vi "NanotecSMCPD.ProcCases.vi"(0 "i ref in":refnum<vi>, 1 "selector":string, 2 "Data":T1, 3 "call cluster":T2={"Object"="", "Selector"="", "CallType"=enum."synchronous", "Async Object"="", "Async Selector"="", "Data Descriptor"="", "Data"=[], "Error #"=0, "Expire"=0}, 5 "error in (no error)":errorcluster) -> (14 "i ref out":refnum<vi>, 17 "answer cluster":T2={"Object"="", "Selector"="", "CallType"=enum."synchronous", "Async Object"="", "Async Selector"="", "Data Descriptor"="", "Data"=[], "Error #"=0, "Expire"=0}, 19 "error out":errorcluster)   [LabVIEW 2014, in "NanotecSMCPD.lvlib"]
doc: "This method is called by a process from within the default case in the event loop. The methods of a class that are linked to events will be called from THIS method. Add your code here."
uses:
  NanotecSMCPD.lvlib
  CS_Core/CSSystem/CoreDefs/CoreDefs.call_type.ctl
  CS_Core/BaseProcess/BaseProcess.descriptor string definition.ctl
  CS_Core/CSSystem/CoreDefs/CoreDefs.rawDataType.ctl
  CS_Core/CSApplicationBaseClasses/MotorBase/MotorBase.statusType.ctl
  CS_Core/CSSystem/CoreLib/CoreLib.string 2 byte array.vi
  CS_Core/CSSystem/CoreLib/CoreLib.short 2 byte array.vi
  CS_Core/CSSystem/CoreLib/CoreLib.byte array 2 int.vi
  CS_Core/CSSystem/CoreLib/CoreLib.int 2 byte array.vi
  CS_Core/CSSystem/CoreLib/CoreLib.double 2 byte array.vi
  CS_Core/CSSystem/CoreLib/CoreLib.byte array 2 double.vi
  CS_Core/CSSystem/CoreLib/CoreLib.byte array 2 short.vi
  CS_Core/CSSystem/CoreLib/CoreLib.lvlib
  CS_Core/BaseProcess/BaseProcess.lvlib
  CS_Core/CSApplicationBaseClasses/MotorBase/MotorBase.lvlib
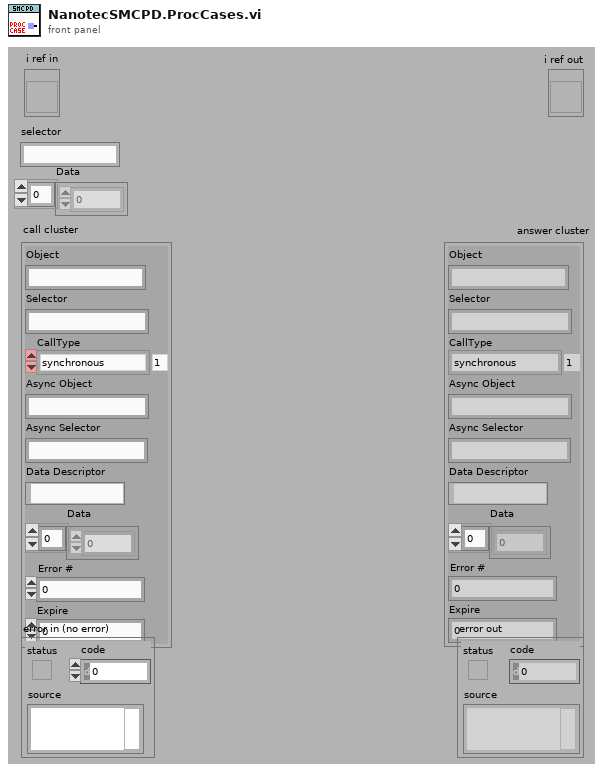
[diagram p1: front panel]
types:
  T1 = typedef "CoreDefs.rawDataType.ctl" = i8[]
  T2 = typedef "CoreDefs.call_type.ctl" = cluster{"Object":string, "Selector":string, "CallType":enum16{"simple", "synchronous", "asynchronous"}, "Async Object":string, "Async Selector":string, "Data Descriptor":T3, "Data":T1, "Error #":i32, "Expire":u32}
  T3 = typedef "BaseProcess.lvlib/BaseProcess.descriptor string definition.ctl" = string
  T4 = typedef "MotorBase.lvlib/MotorBase.statusType.ctl" = u32
  T5 = cluster{"Method":enum16{"MoveRelative", "MoveAbsolute", "Stop"}, "Axis":i32, "Steps":dbl}
  T6 = typedef "NanotecSMCPD.lvlib/NanotecSMCPD.i attribute.ctl" = cluster{"referencing":bool[], "stop":bool[], "AutoHalt ID":i32, "MethodQueue":refnum<queue>, "Referenced1Time?":bool[], "LastCommand ID":i32}
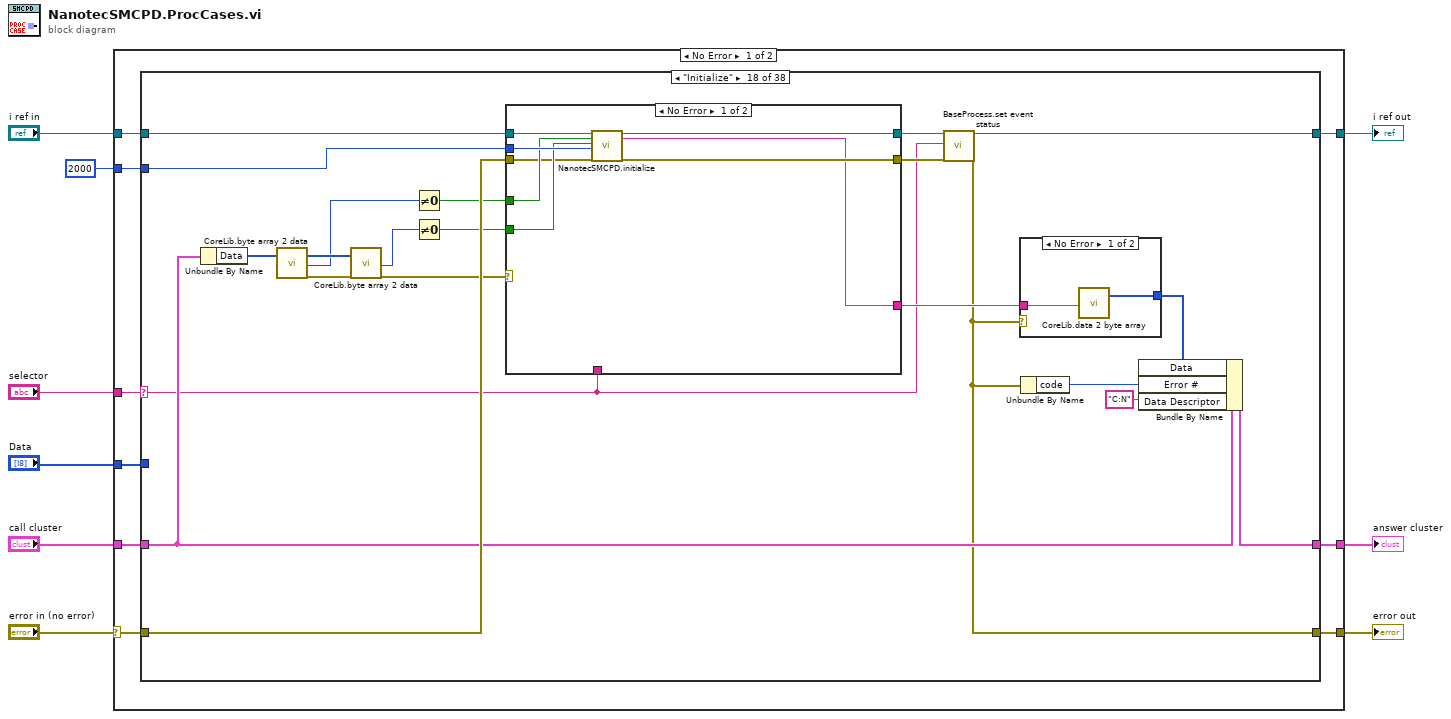
[diagram p0: block diagram]
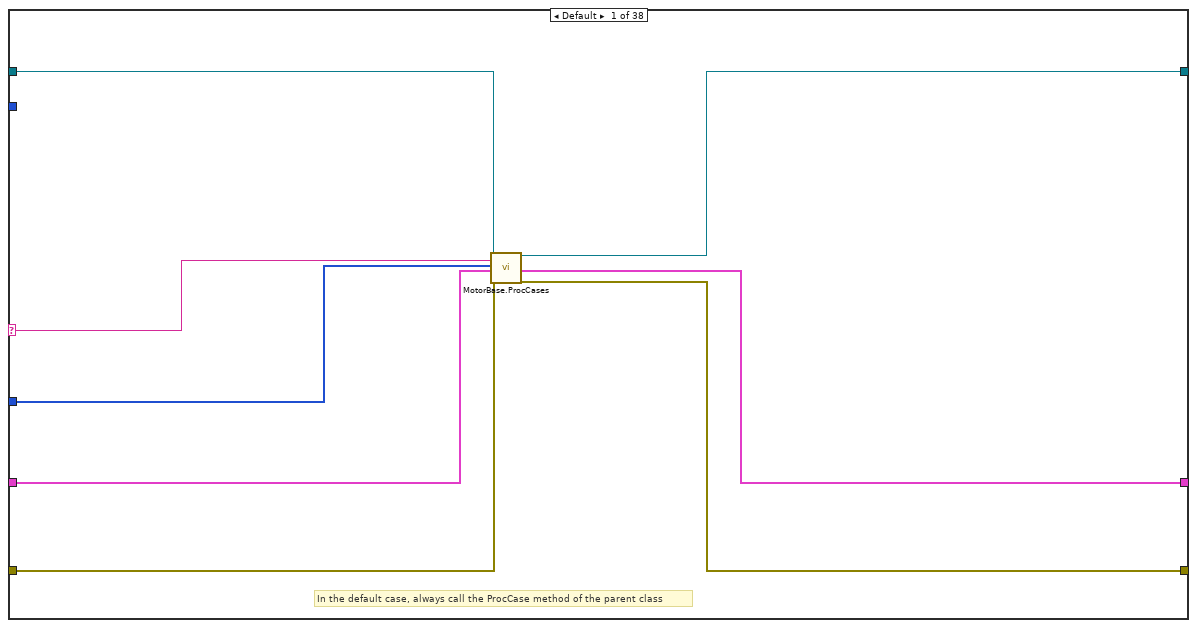
[diagram p2: hidden frame]
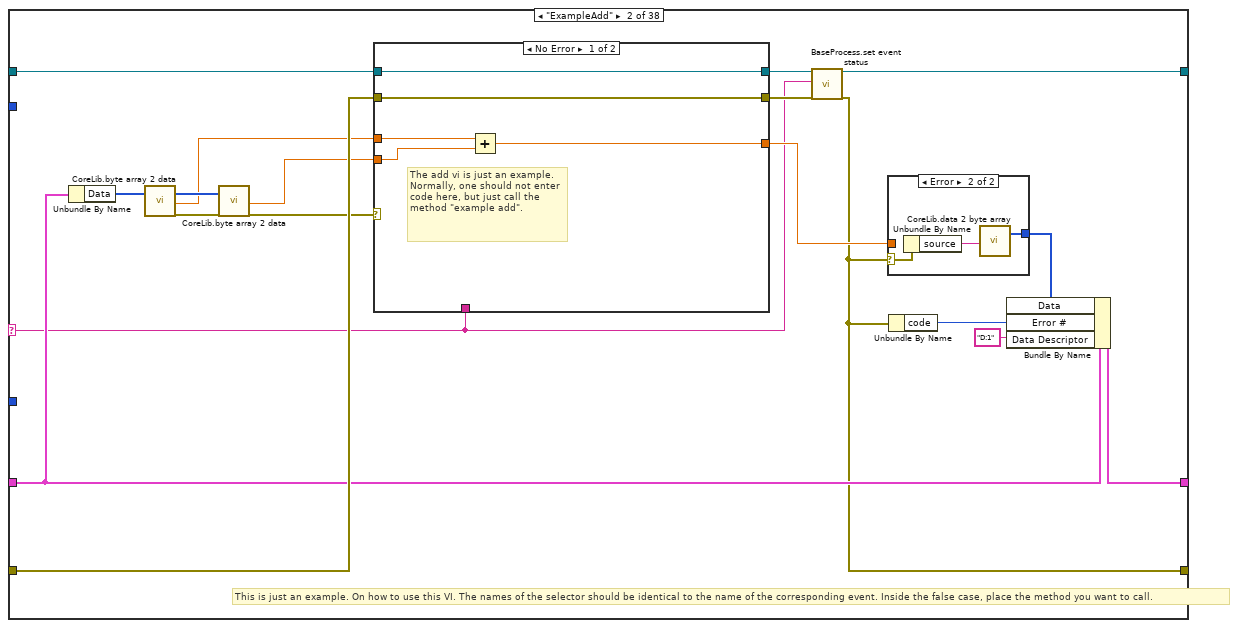
[diagram p3: hidden frame]
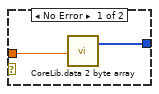
[diagram p4: hidden frame]
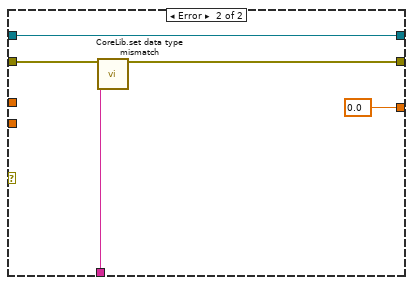
[diagram p5: hidden frame]
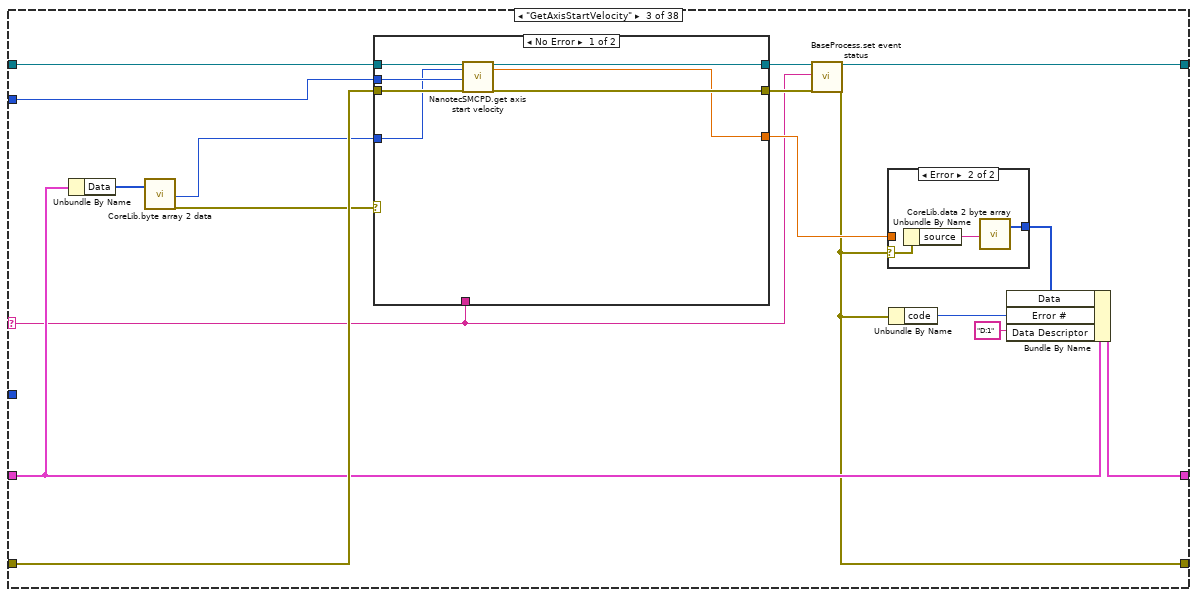
[diagram p6: hidden frame]
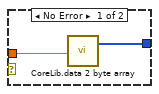
[diagram p7: hidden frame]
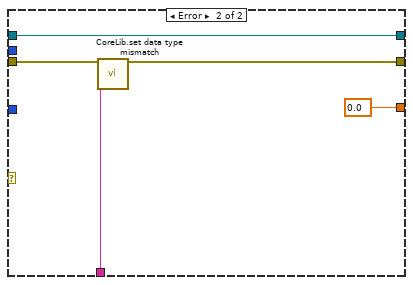
[diagram p8: hidden frame]
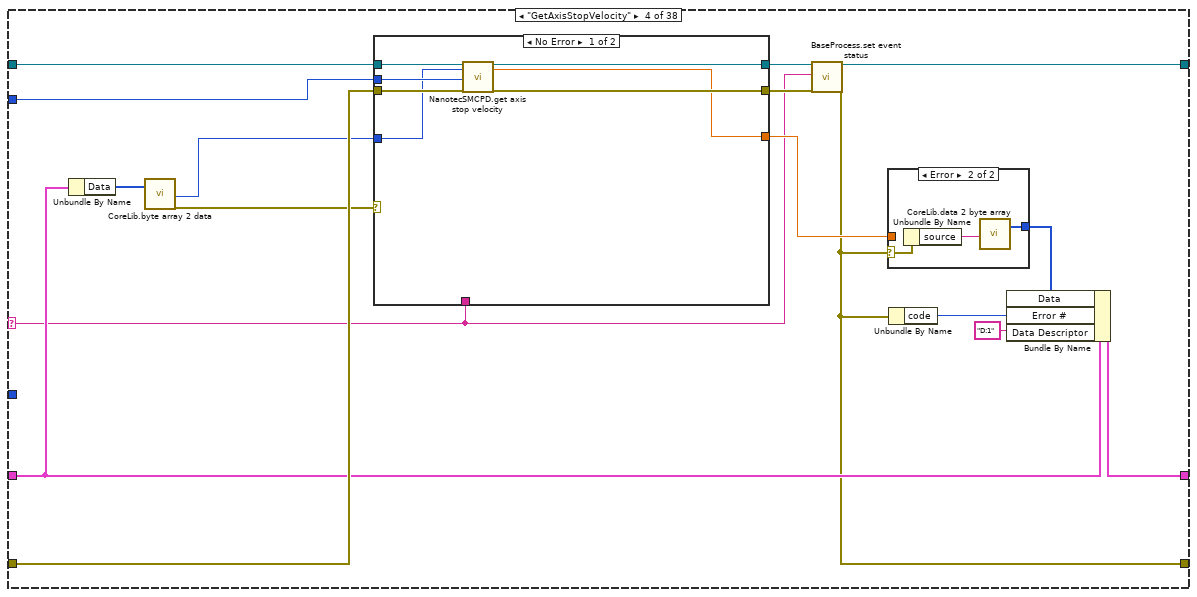
[diagram p9: hidden frame]
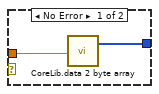
[diagram p10: hidden frame]
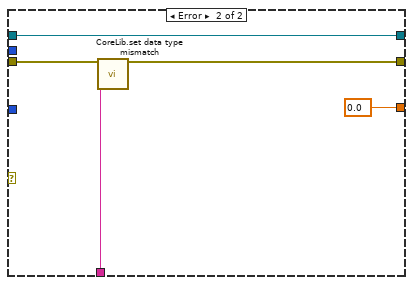
[diagram p11: hidden frame]
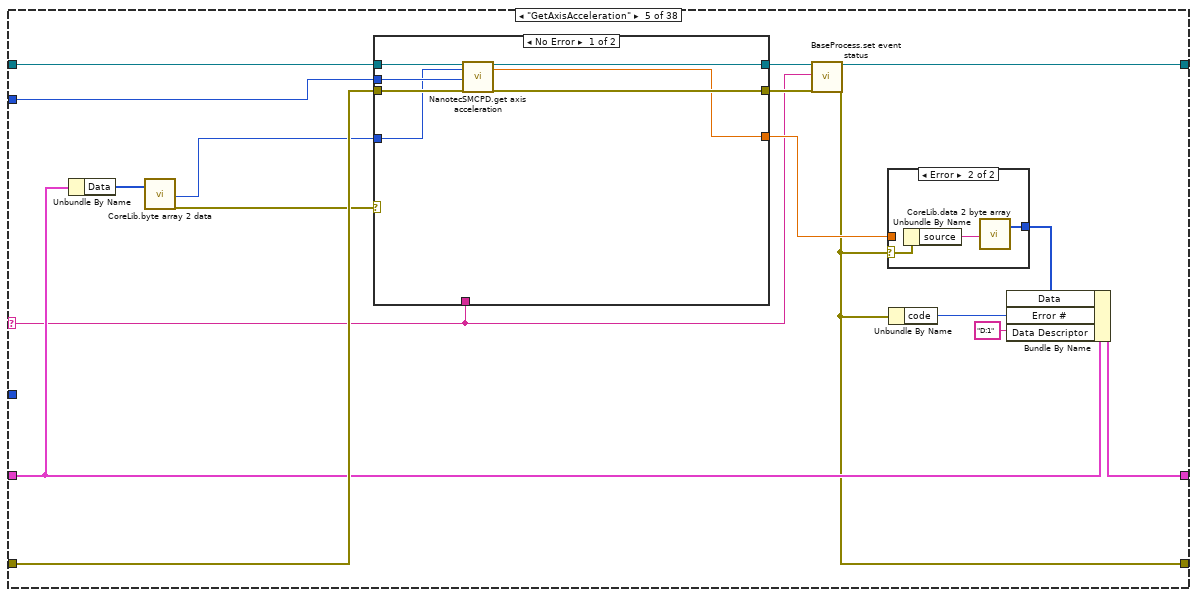
[diagram p12: hidden frame]
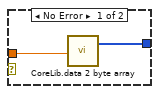
[diagram p13: hidden frame]
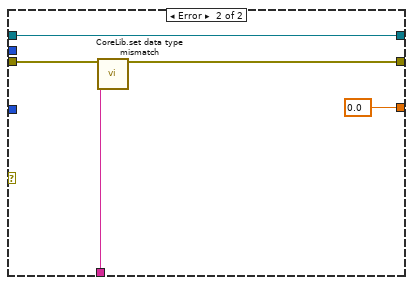
[diagram p14: hidden frame]
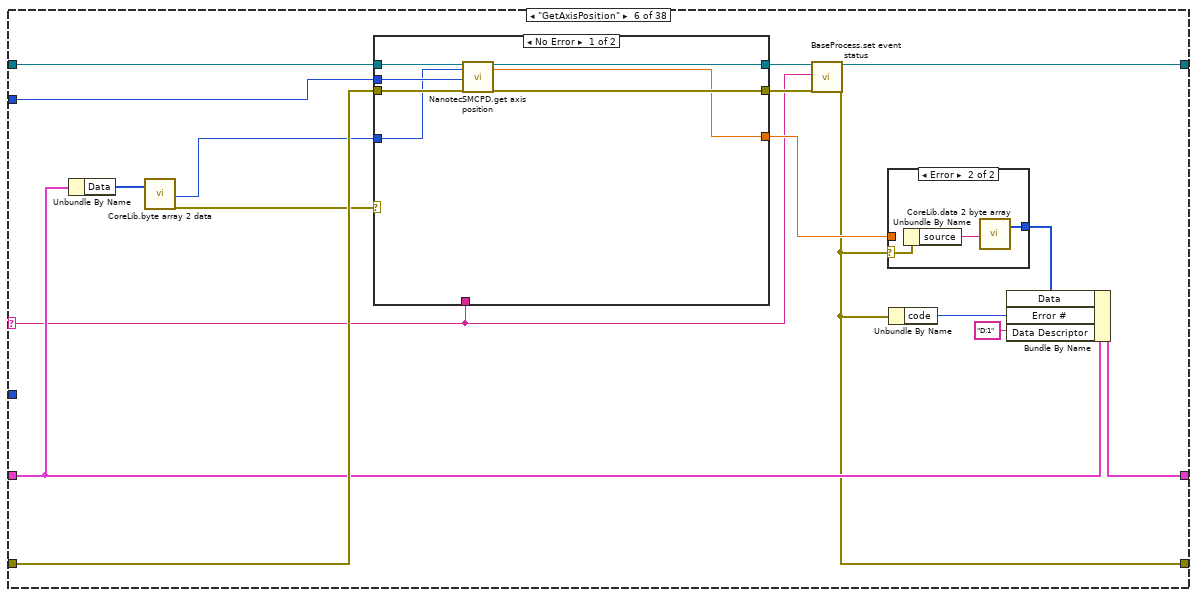
[diagram p15: hidden frame]
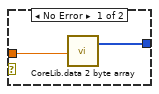
[diagram p16: hidden frame]
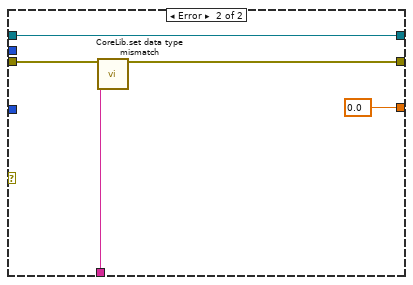
[diagram p17: hidden frame]
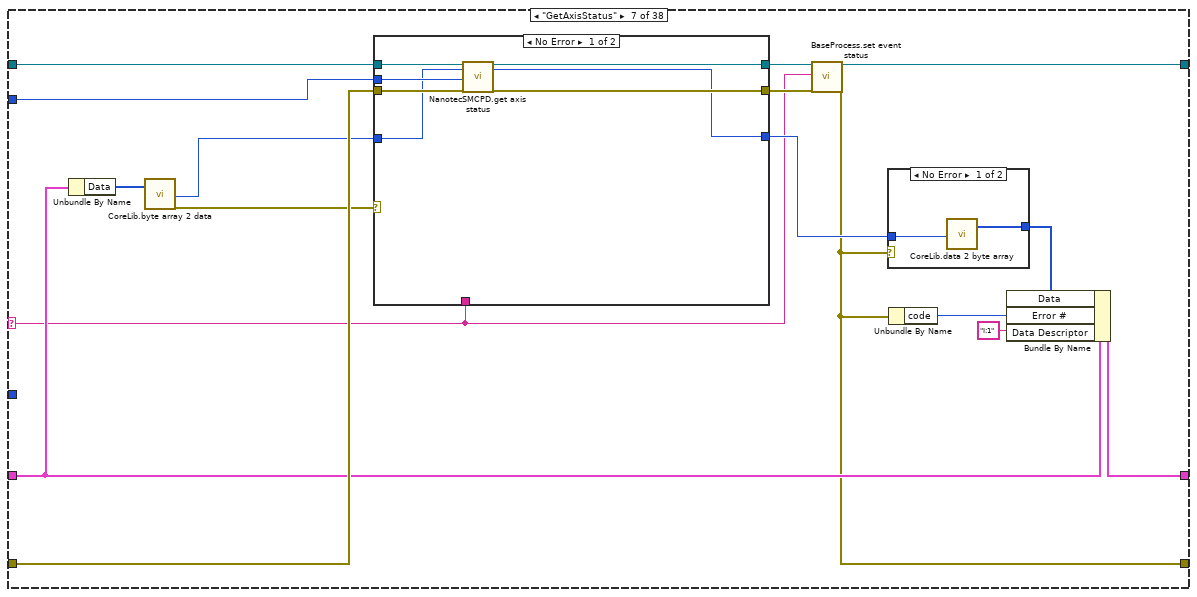
[diagram p18: hidden frame]
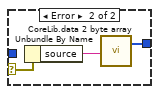
[diagram p19: hidden frame]
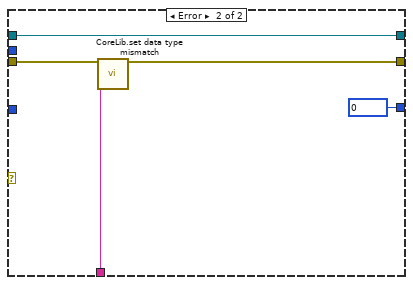
[diagram p20: hidden frame]
diagram:
  n1 = case shown="No Error" "error in (no error)" {
    selector: "error in (no error)" -> [w11 w1067]
    tunnel: "selector" -> [w18 _]
    tunnel: [w17 w1068] -> w8
    tunnel: "Data" -> [w16 _]
    tunnel: "call cluster" -> [w15 w1068]
    tunnel: "i ref in" -> [w14 w1069]
    tunnel: [w13 w1069] -> w4
    tunnel: [w12 w1067] -> w3
    tunnel: 2000 ("ms timeout (10000)") -> [w10 _]
    frame No Error {
      n2 = case shown="\"Initialize\"" w18 {
        selector: w18 -> [w21 w35 w67 w101 w135 w169 w203 w236 w262 w292 w320 w351 w383 w415 w447 w479 w516 w556 w589 w620 w651 w682 w713 w749 w787 w809 w831 w853 w875 w896 w914 w932 w946 w961 w978 w1004 w1018 w1058]
        tunnel: w16 -> [w19 _ _ _ _ _ _ _ _ _ _ _ _ _ _ _ _ _ _ _ _ _ _ _ _ _ _ _ _ _ _ _ _ _ _ _ _ _]
        tunnel: w14 -> [w20 w45 w77 w111 w145 w179 w213 w245 w260 w301 w329 w360 w392 w424 w456 w488 w525 w566 w598 w629 w660 w691 w722 w758 w796 w818 w840 w862 w884 w905 w923 w941 w955 w970 w987 w998 w1023 w1056]
        tunnel: [w26 w34 w66 w100 w134 w168 w202 w235 w259 w291 w319 w350 w382 w414 w446 w478 w515 w555 w588 w619 w650 w681 w712 w748 w786 w808 w830 w852 w874 w895 w913 w931 w945 w960 w977 w1003 w1027 w1057] -> w13
        tunnel: w15 -> [w22 w41 w73 w107 w141 w175 w209 w242 w263 w298 w326 w357 w389 w421 w453 w485 w522 w562 w595 w626 w657 w688 w719 w755 w793 w815 w837 w859 w881 w902 w920 w938 w952 w967 w984 w1010 w1021 w1062]
        tunnel: [w23 w40 w72 w106 w140 w174 w208 w241 w264 w297 w325 w356 w388 w420 w452 w484 w521 w561 w594 w625 w656 w687 w718 w754 w792 w814 w836 w858 w880 w901 w919 w937 w951 w966 w983 w1009 w1032 w1061] -> w17
        tunnel: w11 -> [w25 w44 w76 w110 w144 w178 w212 w244 w266 w300 w328 w359 w391 w423 w455 w487 w524 w565 w597 w628 w659 w690 w721 w757 w795 w817 w839 w861 w883 w904 w922 w940 w954 w969 w986 w995 w1019 w1053]
        tunnel: [w24 w36 w68 w102 w136 w170 w204 w237 w265 w293 w321 w352 w384 w416 w448 w480 w517 w557 w590 w621 w652 w683 w714 w750 w788 w810 w832 w854 w876 w897 w915 w933 w947 w962 w979 w1005 w1028 w1059] -> w12
        tunnel: w10 -> [_ _ w61 w95 w129 w163 w197 w231 w261 w287 w315 w343 w375 w407 w439 w471 w508 w547 w586 w617 w648 w679 w710 w746 w785 w807 w829 w851 w873 w894 w912 w930 _ w959 w976 w993 w1024 w1052]
        frame Default {
          # "In the default case, always call the ProcCase method of the parent class"
          n3 = call "MotorBase.ProcCases.vi"("i ref in"=w20, "selector"=w21, "Data"=w19, "call cluster"=w22, "error in (no error)"=w25) -> ("i ref out"=w26:refnum<vi>, "answer cluster"=w23:T2, "error out"=w24:errorcluster)  [unwired: 12 in]
        }
        frame "ExampleAdd" {
          # "This is just an example. On how to use this VI. The names of the selector should be identical to the name of the corresponding event. Inside the false case, place the method you want to call."
          n4 = Unbundle By Name(w41) -> ("Data"=w32:T1)
          n5 = call-poly "CoreLib.byte array 2 data.vi"("byteArray"=w32) -> ("byteArray out"=w30:T1, "d64"=w28:dbl, "error out"=w31:errorcluster)  [unwired: 16 in]
          n6 = call-poly "CoreLib.byte array 2 data.vi"("byteArray"=w30, "error in (no error)"=w31) -> ("d64"=w27:dbl, "error out"=w29:errorcluster)  [unwired: 15 in, 1 out]
          n7 = case shown="No Error" w29 {
            tunnel: [w52 w60] -> w38
            tunnel: w45 -> [w52 w60]
            tunnel: w44 -> [w53 w59]
            tunnel: [w53 w58] -> w37
            tunnel: w27 -> [w55 _]
            tunnel: [w54 0.0] -> w43
            tunnel: w35 -> [_ w56]
            tunnel: w28 -> [w51 _]
            frame No Error {
              # "The add vi is just an example. Normally, one should not enter code here, but just call the method \"example add\"."
              n8 = Add(x=w51, y=w55) -> (x+y=w54:dbl)
            }
            frame Error {
              n9 = call "CoreLib.set data type mismatch.vi"("error in (no error)"=w59, "error source"=w56) -> ("error out"=w58:errorcluster)  [unwired: 17 in]
            }
          }
          n10 = call "BaseProcess.set event status.vi"("i ref in"=w38, "EventStatus"=w35, "error in (no error)"=w37) -> ("i ref out"=w34:refnum<vi>, "error out"=w36:errorcluster)  [unwired: 14 in, 1 out]
          n11 = case shown="Error" w36 {
            selector: w36 -> [_ w50]
            tunnel: [w46 w49] -> w39
            tunnel: w43 -> [w47 _]
            frame No Error {
              n12 = call-poly "CoreLib.data 2 byte array.vi"("f64"=w47) -> ("byteArray out"=w46:T1)  [unwired: 18 in]
            }
            frame Error {
              n13 = Unbundle By Name(w50) -> ("source"=w48:string)
              n14 = call-poly "CoreLib.data 2 byte array.vi"("string"=w48) -> ("byteArray out"=w49:T1)  [unwired: 18 in]
            }
          }
          n15 = Unbundle By Name(w36) -> ("code"=w42:i32)
          n16 = Bundle By Name(cluster=w41, "Data"=w39, "Error #"=w42, "Data Descriptor"="D:1") -> (w40:T2)
        }
        frame "GetAxisStartVelocity" {
          n17 = Unbundle By Name(w73) -> ("Data"=w64:T1)
          n18 = call-poly "CoreLib.byte array 2 data.vi"("byteArray"=w64) -> ("i32"=w63:i32, "error out"=w62:errorcluster)  [unwired: 16 in, 1 out]
          n19 = case shown="No Error" w62 {
            tunnel: [w88 w94] -> w70
            tunnel: w77 -> [w89 w94]
            tunnel: w76 -> [w86 w93]
            tunnel: [w87 w92] -> w69
            tunnel: [w83 0.0] -> w75
            tunnel: w67 -> [_ w90]
            tunnel: w63 -> [w84 _]
            tunnel: w61 -> [w85 _]
            frame No Error {
              n20 = call "NanotecSMCPD.get axis start velocity.vi"("i ref in"=w89, "axis"=w84, "ms timeout (10000)"=w85, "error in (no error)"=w86) -> ("i ref out"=w88:refnum<vi>, "startVelocity [unit/s]"=w83:dbl, "error out"=w87:errorcluster)  [unwired: 12 in, 1 out]
            }
            frame Error {
              n21 = call "CoreLib.set data type mismatch.vi"("error in (no error)"=w93, "error source"=w90) -> ("error out"=w92:errorcluster)  [unwired: 17 in]
            }
          }
          n22 = call "BaseProcess.set event status.vi"("i ref in"=w70, "EventStatus"=w67, "error in (no error)"=w69) -> ("i ref out"=w66:refnum<vi>, "error out"=w68:errorcluster)  [unwired: 14 in, 1 out]
          n23 = case shown="Error" w68 {
            selector: w68 -> [_ w82]
            tunnel: [w78 w81] -> w71
            tunnel: w75 -> [w79 _]
            frame No Error {
              n24 = call-poly "CoreLib.data 2 byte array.vi"("f64"=w79) -> ("byteArray out"=w78:T1)  [unwired: 18 in]
            }
            frame Error {
              n25 = Unbundle By Name(w82) -> ("source"=w80:string)
              n26 = call-poly "CoreLib.data 2 byte array.vi"("string"=w80) -> ("byteArray out"=w81:T1)  [unwired: 18 in]
            }
          }
          n27 = Unbundle By Name(w68) -> ("code"=w74:i32)
          n28 = Bundle By Name(cluster=w73, "Data"=w71, "Error #"=w74, "Data Descriptor"="D:1") -> (w72:T2)
        }
        frame "GetAxisStopVelocity" {
          n29 = Unbundle By Name(w107) -> ("Data"=w98:T1)
          n30 = call-poly "CoreLib.byte array 2 data.vi"("byteArray"=w98) -> ("i32"=w97:i32, "error out"=w96:errorcluster)  [unwired: 16 in, 1 out]
          n31 = case shown="No Error" w96 {
            tunnel: [w122 w128] -> w104
            tunnel: w111 -> [w123 w128]
            tunnel: w110 -> [w120 w127]
            tunnel: [w121 w126] -> w103
            tunnel: [w117 0.0] -> w109
            tunnel: w101 -> [_ w124]
            tunnel: w97 -> [w118 _]
            tunnel: w95 -> [w119 _]
            frame No Error {
              n32 = call "NanotecSMCPD.get axis stop velocity.vi"("i ref in"=w123, "axis"=w118, "ms timeout (10000)"=w119, "error in (no error)"=w120) -> ("i ref out"=w122:refnum<vi>, "stopVelocity [unit/s]"=w117:dbl, "error out"=w121:errorcluster)  [unwired: 12 in, 1 out]
            }
            frame Error {
              n33 = call "CoreLib.set data type mismatch.vi"("error in (no error)"=w127, "error source"=w124) -> ("error out"=w126:errorcluster)  [unwired: 17 in]
            }
          }
          n34 = call "BaseProcess.set event status.vi"("i ref in"=w104, "EventStatus"=w101, "error in (no error)"=w103) -> ("i ref out"=w100:refnum<vi>, "error out"=w102:errorcluster)  [unwired: 14 in, 1 out]
          n35 = case shown="Error" w102 {
            selector: w102 -> [_ w116]
            tunnel: [w112 w115] -> w105
            tunnel: w109 -> [w113 _]
            frame No Error {
              n36 = call-poly "CoreLib.data 2 byte array.vi"("f64"=w113) -> ("byteArray out"=w112:T1)  [unwired: 18 in]
            }
            frame Error {
              n37 = Unbundle By Name(w116) -> ("source"=w114:string)
              n38 = call-poly "CoreLib.data 2 byte array.vi"("string"=w114) -> ("byteArray out"=w115:T1)  [unwired: 18 in]
            }
          }
          n39 = Unbundle By Name(w102) -> ("code"=w108:i32)
          n40 = Bundle By Name(cluster=w107, "Data"=w105, "Error #"=w108, "Data Descriptor"="D:1") -> (w106:T2)
        }
        frame "GetAxisAcceleration" {
          n41 = Unbundle By Name(w141) -> ("Data"=w132:T1)
          n42 = call-poly "CoreLib.byte array 2 data.vi"("byteArray"=w132) -> ("i32"=w131:i32, "error out"=w130:errorcluster)  [unwired: 16 in, 1 out]
          n43 = case shown="No Error" w130 {
            tunnel: [w156 w162] -> w138
            tunnel: w145 -> [w157 w162]
            tunnel: w144 -> [w154 w161]
            tunnel: [w155 w160] -> w137
            tunnel: [w151 0.0] -> w143
            tunnel: w135 -> [_ w158]
            tunnel: w131 -> [w152 _]
            tunnel: w129 -> [w153 _]
            frame No Error {
              n44 = call "NanotecSMCPD.get axis acceleration.vi"("i ref in"=w157, "axis"=w152, "ms timeout (10000)"=w153, "error in (no error)"=w154) -> ("i ref out"=w156:refnum<vi>, "acceleration [unit/s^2]"=w151:dbl, "error out"=w155:errorcluster)  [unwired: 12 in, 1 out]
            }
            frame Error {
              n45 = call "CoreLib.set data type mismatch.vi"("error in (no error)"=w161, "error source"=w158) -> ("error out"=w160:errorcluster)  [unwired: 17 in]
            }
          }
          n46 = call "BaseProcess.set event status.vi"("i ref in"=w138, "EventStatus"=w135, "error in (no error)"=w137) -> ("i ref out"=w134:refnum<vi>, "error out"=w136:errorcluster)  [unwired: 14 in, 1 out]
          n47 = case shown="Error" w136 {
            selector: w136 -> [_ w150]
            tunnel: [w146 w149] -> w139
            tunnel: w143 -> [w147 _]
            frame No Error {
              n48 = call-poly "CoreLib.data 2 byte array.vi"("f64"=w147) -> ("byteArray out"=w146:T1)  [unwired: 18 in]
            }
            frame Error {
              n49 = Unbundle By Name(w150) -> ("source"=w148:string)
              n50 = call-poly "CoreLib.data 2 byte array.vi"("string"=w148) -> ("byteArray out"=w149:T1)  [unwired: 18 in]
            }
          }
          n51 = Unbundle By Name(w136) -> ("code"=w142:i32)
          n52 = Bundle By Name(cluster=w141, "Data"=w139, "Error #"=w142, "Data Descriptor"="D:1") -> (w140:T2)
        }
        frame "GetAxisPosition" {
          n53 = Unbundle By Name(w175) -> ("Data"=w166:T1)
          n54 = call-poly "CoreLib.byte array 2 data.vi"("byteArray"=w166) -> ("i32"=w165:i32, "error out"=w164:errorcluster)  [unwired: 16 in, 1 out]
          n55 = case shown="No Error" w164 {
            tunnel: [w190 w196] -> w172
            tunnel: w179 -> [w191 w196]
            tunnel: w178 -> [w188 w195]
            tunnel: [w189 w194] -> w171
            tunnel: [w185 0.0] -> w177
            tunnel: w169 -> [_ w192]
            tunnel: w165 -> [w186 _]
            tunnel: w163 -> [w187 _]
            frame No Error {
              n56 = call "NanotecSMCPD.get axis position.vi"("i ref in"=w191, "axis"=w186, "ms timeout (10000)"=w187, "error in (no error)"=w188) -> ("i ref out"=w190:refnum<vi>, "position [unit]"=w185:dbl, "error out"=w189:errorcluster)  [unwired: 12 in, 1 out]
            }
            frame Error {
              n57 = call "CoreLib.set data type mismatch.vi"("error in (no error)"=w195, "error source"=w192) -> ("error out"=w194:errorcluster)  [unwired: 17 in]
            }
          }
          n58 = call "BaseProcess.set event status.vi"("i ref in"=w172, "EventStatus"=w169, "error in (no error)"=w171) -> ("i ref out"=w168:refnum<vi>, "error out"=w170:errorcluster)  [unwired: 14 in, 1 out]
          n59 = case shown="Error" w170 {
            selector: w170 -> [_ w184]
            tunnel: [w180 w183] -> w173
            tunnel: w177 -> [w181 _]
            frame No Error {
              n60 = call-poly "CoreLib.data 2 byte array.vi"("f64"=w181) -> ("byteArray out"=w180:T1)  [unwired: 18 in]
            }
            frame Error {
              n61 = Unbundle By Name(w184) -> ("source"=w182:string)
              n62 = call-poly "CoreLib.data 2 byte array.vi"("string"=w182) -> ("byteArray out"=w183:T1)  [unwired: 18 in]
            }
          }
          n63 = Unbundle By Name(w170) -> ("code"=w176:i32)
          n64 = Bundle By Name(cluster=w175, "Data"=w173, "Error #"=w176, "Data Descriptor"="D:1") -> (w174:T2)
        }
        frame "GetAxisStatus" {
          n65 = Unbundle By Name(w209) -> ("Data"=w200:T1)
          n66 = call-poly "CoreLib.byte array 2 data.vi"("byteArray"=w200) -> ("i32"=w199:i32, "error out"=w198:errorcluster)  [unwired: 16 in, 1 out]
          n67 = case shown="No Error" w198 {
            tunnel: [w224 w230] -> w206
            tunnel: w213 -> [w225 w230]
            tunnel: w212 -> [w222 w229]
            tunnel: [w223 w228] -> w205
            tunnel: [w219 w226] -> w211
            tunnel: w203 -> [_ w227]
            tunnel: w199 -> [w220 _]
            tunnel: w197 -> [w221 _]
            frame No Error {
              n68 = call "NanotecSMCPD.get axis status.vi"("i ref in"=w225, "axis"=w220, "ms timeout (10000)"=w221, "error in (no error)"=w222) -> ("i ref out"=w224:refnum<vi>, "status"=w219:T4, "error out"=w223:errorcluster)  [unwired: 11 in, 2 out]
            }
            frame Error {
              w226 = T4 0 items=["motorEnabled"=1, "negativeLimitSwitchActive"=2, "positiveLimitSwitchActive"=4, "limitSwitchesEnabled"=8, "limitSwitchesAreNormallyClosed"=16, "reseved1"=32, "referenced"=64, "inPosition"=128, "reserved2"=256, "reserved3"=512, "reserved4"=1024, "reserved5"=2048, "error"=4096, "reserved6"=8192, "reserved7"=16384, "reserved8"=32768, "user defined1"=65536, "user defined2"=131072, "user defined3"=262144, "user defined4"=524288, "user defined5"=1048576, "user defined6"=2097152, "user defined7"=4194304, "user defined8"=8388608, "user defined9"=16777216, "user defined10"=33554432, "user defined11"=67108864, "user defined12"=134217728, "user defined13"=268435456, "user defined14"=536870912, "user defined15"=1073741824, "user defined16"=2147483648] ("status")
              n69 = call "CoreLib.set data type mismatch.vi"("error in (no error)"=w229, "error source"=w227) -> ("error out"=w228:errorcluster)  [unwired: 17 in]
            }
          }
          n70 = call "BaseProcess.set event status.vi"("i ref in"=w206, "EventStatus"=w203, "error in (no error)"=w205) -> ("i ref out"=w202:refnum<vi>, "error out"=w204:errorcluster)  [unwired: 14 in, 1 out]
          n71 = case shown="No Error" w204 {
            selector: w204 -> [_ w218]
            tunnel: [w214 w217] -> w207
            tunnel: w211 -> [w215 _]
            frame No Error {
              n72 = call-poly "CoreLib.data 2 byte array.vi"("i32"=w215) -> ("byteArray out"=w214:T1)  [unwired: 18 in]
            }
            frame Error {
              n73 = Unbundle By Name(w218) -> ("source"=w216:string)
              n74 = call-poly "CoreLib.data 2 byte array.vi"("string"=w216) -> ("byteArray out"=w217:T1)  [unwired: 18 in]
            }
          }
          n75 = Unbundle By Name(w204) -> ("code"=w210:i32)
          n76 = Bundle By Name(cluster=w209, "Data"=w207, "Error #"=w210, "Data Descriptor"="I:1") -> (w208:T2)
        }
        frame "ResetAxis" {
          n77 = Unbundle By Name(w242) -> ("Data"=w234:T1)
          n78 = call-poly "CoreLib.byte array 2 data.vi"("byteArray"=w234) -> ("i32"=w233:i32, "error out"=w232:errorcluster)  [unwired: 16 in, 1 out]
          n79 = case shown="No Error" w232 {
            tunnel: [w253 w258] -> w239
            tunnel: w245 -> [w254 w258]
            tunnel: w244 -> [w251 w257]
            tunnel: [w252 w256] -> w238
            tunnel: w236 -> [_ w255]
            tunnel: w233 -> [w249 _]
            tunnel: w231 -> [w250 _]
            frame No Error {
              n80 = call "NanotecSMCPD.reset axis.vi"("i ref in"=w254, "axis"=w249, "ms timeout (10000)"=w250, "error in (no error)"=w251) -> ("i ref out"=w253:refnum<vi>, "error out"=w252:errorcluster)  [unwired: 13 in, 1 out]
            }
            frame Error {
              n81 = call "CoreLib.set data type mismatch.vi"("error in (no error)"=w257, "error source"=w255) -> ("error out"=w256:errorcluster)  [unwired: 17 in]
            }
          }
          n82 = call "BaseProcess.set event status.vi"("i ref in"=w239, "EventStatus"=w236, "error in (no error)"=w238) -> ("i ref out"=w235:refnum<vi>, "error out"=w237:errorcluster)  [unwired: 14 in, 1 out]
          n83 = case shown="No Error" w237 {
            selector: w237 -> [_ w248]
            tunnel: [_ w247] -> w240
            frame No Error {
            }
            frame Error {
              n84 = Unbundle By Name(w248) -> ("source"=w246:string)
              n85 = call-poly "CoreLib.data 2 byte array.vi"("string"=w246) -> ("byteArray out"=w247:T1)  [unwired: 18 in]
            }
          }
          n86 = Unbundle By Name(w237) -> ("code"=w243:i32)
          n87 = Bundle By Name(cluster=w242, "Data"=w240, "Error #"=w243) -> (w241:T2)
        }
        frame "ResetPositionError" {
          n88 = Unbundle By Name(w263) -> ("Data"=w269:T1)
          n89 = call-poly "CoreLib.byte array 2 data.vi"("byteArray"=w269) -> ("i32"=w268:i32, "error out"=w267:errorcluster)  [unwired: 16 in, 1 out]
          n90 = case shown="No Error" w267 {
            tunnel: [w281 w286] -> w271
            tunnel: w260 -> [w282 w286]
            tunnel: w266 -> [w279 w285]
            tunnel: [w280 w284] -> w270
            tunnel: w262 -> [_ w283]
            tunnel: w268 -> [w277 _]
            tunnel: w261 -> [w278 _]
            frame No Error {
              n91 = call "NanotecSMCPD.reset axis position error.vi"("i ref in"=w282, "axis"=w277, "ms timeout (10000)"=w278, "error in (no error)"=w279) -> ("i ref out"=w281:refnum<vi>, "error out"=w280:errorcluster)  [unwired: 14 in]
            }
            frame Error {
              n92 = call "CoreLib.set data type mismatch.vi"("error in (no error)"=w285, "error source"=w283) -> ("error out"=w284:errorcluster)  [unwired: 17 in]
            }
          }
          n93 = call "BaseProcess.set event status.vi"("i ref in"=w271, "EventStatus"=w262, "error in (no error)"=w270) -> ("i ref out"=w259:refnum<vi>, "error out"=w265:errorcluster)  [unwired: 14 in, 1 out]
          n94 = case shown="No Error" w265 {
            selector: w265 -> [_ w276]
            tunnel: [_ w275] -> w272
            frame No Error {
            }
            frame Error {
              n95 = Unbundle By Name(w276) -> ("source"=w274:string)
              n96 = call-poly "CoreLib.data 2 byte array.vi"("string"=w274) -> ("byteArray out"=w275:T1)  [unwired: 18 in]
            }
          }
          n97 = Unbundle By Name(w265) -> ("code"=w273:i32)
          n98 = Bundle By Name(cluster=w263, "Data"=w272, "Error #"=w273) -> (w264:T2)
        }
        frame "HaltAxis" {
          n99 = Unbundle By Name(w298) -> ("Data"=w290:T1)
          n100 = call-poly "CoreLib.byte array 2 data.vi"("byteArray"=w290) -> ("i32"=w289:i32, "error out"=w288:errorcluster)  [unwired: 16 in, 1 out]
          n101 = case shown="No Error" w288 {
            tunnel: [w309 w314] -> w295
            tunnel: w301 -> [w310 w314]
            tunnel: w300 -> [w307 w313]
            tunnel: [w308 w312] -> w294
            tunnel: w292 -> [_ w311]
            tunnel: w289 -> [w305 _]
            tunnel: w287 -> [w306 _]
            frame No Error {
              n102 = call "NanotecSMCPD.halt axis.vi"("i ref in"=w310, "axis"=w305, "ms timeout (10000)"=w306, "error in (no error)"=w307) -> ("i ref out"=w309:refnum<vi>, "error out"=w308:errorcluster)  [unwired: 13 in, 1 out]
            }
            frame Error {
              n103 = call "CoreLib.set data type mismatch.vi"("error in (no error)"=w313, "error source"=w311) -> ("error out"=w312:errorcluster)  [unwired: 17 in]
            }
          }
          n104 = call "BaseProcess.set event status.vi"("i ref in"=w295, "EventStatus"=w292, "error in (no error)"=w294) -> ("i ref out"=w291:refnum<vi>, "error out"=w293:errorcluster)  [unwired: 14 in, 1 out]
          n105 = case shown="No Error" w293 {
            selector: w293 -> [_ w304]
            tunnel: [_ w303] -> w296
            frame No Error {
            }
            frame Error {
              n106 = Unbundle By Name(w304) -> ("source"=w302:string)
              n107 = call-poly "CoreLib.data 2 byte array.vi"("string"=w302) -> ("byteArray out"=w303:T1)  [unwired: 18 in]
            }
          }
          n108 = Unbundle By Name(w293) -> ("code"=w299:i32)
          n109 = Bundle By Name(cluster=w298, "Data"=w296, "Error #"=w299) -> (w297:T2)
        }
        frame "FindAxisReference" {
          n110 = Unbundle By Name(w326) -> ("Data"=w318:T1)
          n111 = call-poly "CoreLib.byte array 2 data.vi"("byteArray"=w318) -> ("i32"=w317:i32, "error out"=w316:errorcluster)  [unwired: 16 in, 1 out]
          n112 = case shown="No Error" w316 {
            tunnel: [w337 w342] -> w323
            tunnel: w329 -> [w338 w342]
            tunnel: w328 -> [w335 w341]
            tunnel: [w336 w340] -> w322
            tunnel: w320 -> [_ w339]
            tunnel: w317 -> [w333 _]
            tunnel: w315 -> [w334 _]
            frame No Error {
              n113 = call "NanotecSMCPD.find axis reference.vi"("i ref in"=w338, "axis"=w333, "ms timeout (10000)"=w334, "error in (no error)"=w335) -> ("i ref out"=w337:refnum<vi>, "error out"=w336:errorcluster)  [unwired: 13 in, 1 out]
            }
            frame Error {
              n114 = call "CoreLib.set data type mismatch.vi"("error in (no error)"=w341, "error source"=w339) -> ("error out"=w340:errorcluster)  [unwired: 17 in]
            }
          }
          n115 = call "BaseProcess.set event status.vi"("i ref in"=w323, "EventStatus"=w320, "error in (no error)"=w322) -> ("i ref out"=w319:refnum<vi>, "error out"=w321:errorcluster)  [unwired: 14 in, 1 out]
          n116 = case shown="No Error" w321 {
            selector: w321 -> [_ w332]
            tunnel: [_ w331] -> w324
            frame No Error {
            }
            frame Error {
              n117 = Unbundle By Name(w332) -> ("source"=w330:string)
              n118 = call-poly "CoreLib.data 2 byte array.vi"("string"=w330) -> ("byteArray out"=w331:T1)  [unwired: 18 in]
            }
          }
          n119 = Unbundle By Name(w321) -> ("code"=w327:i32)
          n120 = Bundle By Name(cluster=w326, "Data"=w324, "Error #"=w327) -> (w325:T2)
        }
        frame "SetAxisStartVelocity" {
          n121 = Unbundle By Name(w357) -> ("Data"=w349:T1)
          n122 = call-poly "CoreLib.byte array 2 data.vi"("byteArray"=w349) -> ("byteArray out"=w347:T1, "i32"=w345:i32, "error out"=w348:errorcluster)  [unwired: 16 in]
          n123 = call-poly "CoreLib.byte array 2 data.vi"("byteArray"=w347, "error in (no error)"=w348) -> ("d64"=w344:dbl, "error out"=w346:errorcluster)  [unwired: 15 in, 1 out]
          n124 = case shown="No Error" w346 {
            tunnel: [w367 w374] -> w354
            tunnel: w360 -> [w370 w374]
            tunnel: w359 -> [w369 w373]
            tunnel: [w368 w372] -> w353
            tunnel: w344 -> [w365 _]
            tunnel: w351 -> [_ w371]
            tunnel: w345 -> [w366 _]
            tunnel: w343 -> [w364 _]
            frame No Error {
              n125 = call "NanotecSMCPD.set axis start velocity.vi"("i ref in"=w370, "axis"=w366, "velocity [units/s]"=w365, "ms timeout (10000)"=w364, "error in (no error)"=w369) -> ("i ref out"=w367:refnum<vi>, "error out"=w368:errorcluster)  [unwired: 12 in, 1 out]
            }
            frame Error {
              n126 = call "CoreLib.set data type mismatch.vi"("error in (no error)"=w373, "error source"=w371) -> ("error out"=w372:errorcluster)  [unwired: 17 in]
            }
          }
          n127 = call "BaseProcess.set event status.vi"("i ref in"=w354, "EventStatus"=w351, "error in (no error)"=w353) -> ("i ref out"=w350:refnum<vi>, "error out"=w352:errorcluster)  [unwired: 14 in, 1 out]
          n128 = case shown="No Error" w352 {
            selector: w352 -> [_ w363]
            tunnel: [_ w362] -> w355
            frame No Error {
            }
            frame Error {
              n129 = Unbundle By Name(w363) -> ("source"=w361:string)
              n130 = call-poly "CoreLib.data 2 byte array.vi"("string"=w361) -> ("byteArray out"=w362:T1)  [unwired: 18 in]
            }
          }
          n131 = Unbundle By Name(w352) -> ("code"=w358:i32)
          n132 = Bundle By Name(cluster=w357, "Data"=w355, "Error #"=w358) -> (w356:T2)
        }
        frame "SetAxisStopVelocity" {
          n133 = Unbundle By Name(w389) -> ("Data"=w381:T1)
          n134 = call-poly "CoreLib.byte array 2 data.vi"("byteArray"=w381) -> ("byteArray out"=w379:T1, "i32"=w377:i32, "error out"=w380:errorcluster)  [unwired: 16 in]
          n135 = call-poly "CoreLib.byte array 2 data.vi"("byteArray"=w379, "error in (no error)"=w380) -> ("d64"=w376:dbl, "error out"=w378:errorcluster)  [unwired: 15 in, 1 out]
          n136 = case shown="No Error" w378 {
            tunnel: [w399 w406] -> w386
            tunnel: w392 -> [w402 w406]
            tunnel: w391 -> [w401 w405]
            tunnel: [w400 w404] -> w385
            tunnel: w376 -> [w397 _]
            tunnel: w383 -> [_ w403]
            tunnel: w377 -> [w398 _]
            tunnel: w375 -> [w396 _]
            frame No Error {
              n137 = call "NanotecSMCPD.set axis stop velocity.vi"("i ref in"=w402, "axis"=w398, "velocity [units/s]"=w397, "ms timeout (10000)"=w396, "error in (no error)"=w401) -> ("i ref out"=w399:refnum<vi>, "error out"=w400:errorcluster)  [unwired: 12 in, 1 out]
            }
            frame Error {
              n138 = call "CoreLib.set data type mismatch.vi"("error in (no error)"=w405, "error source"=w403) -> ("error out"=w404:errorcluster)  [unwired: 17 in]
            }
          }
          n139 = call "BaseProcess.set event status.vi"("i ref in"=w386, "EventStatus"=w383, "error in (no error)"=w385) -> ("i ref out"=w382:refnum<vi>, "error out"=w384:errorcluster)  [unwired: 14 in, 1 out]
          n140 = case shown="No Error" w384 {
            selector: w384 -> [_ w395]
            tunnel: [_ w394] -> w387
            frame No Error {
            }
            frame Error {
              n141 = Unbundle By Name(w395) -> ("source"=w393:string)
              n142 = call-poly "CoreLib.data 2 byte array.vi"("string"=w393) -> ("byteArray out"=w394:T1)  [unwired: 18 in]
            }
          }
          n143 = Unbundle By Name(w384) -> ("code"=w390:i32)
          n144 = Bundle By Name(cluster=w389, "Data"=w387, "Error #"=w390) -> (w388:T2)
        }
        frame "SetAxisAcceleration" {
          n145 = Unbundle By Name(w421) -> ("Data"=w413:T1)
          n146 = call-poly "CoreLib.byte array 2 data.vi"("byteArray"=w413) -> ("byteArray out"=w411:T1, "i32"=w409:i32, "error out"=w412:errorcluster)  [unwired: 16 in]
          n147 = call-poly "CoreLib.byte array 2 data.vi"("byteArray"=w411, "error in (no error)"=w412) -> ("d64"=w408:dbl, "error out"=w410:errorcluster)  [unwired: 15 in, 1 out]
          n148 = case shown="No Error" w410 {
            tunnel: [w431 w438] -> w418
            tunnel: w424 -> [w434 w438]
            tunnel: w423 -> [w433 w437]
            tunnel: [w432 w436] -> w417
            tunnel: w408 -> [w429 _]
            tunnel: w415 -> [_ w435]
            tunnel: w409 -> [w430 _]
            tunnel: w407 -> [w428 _]
            frame No Error {
              n149 = call "NanotecSMCPD.set axis acceleration.vi"("i ref in"=w434, "axis"=w430, "acceleration [unit/s^2]"=w429, "ms timeout (10000)"=w428, "error in (no error)"=w433) -> ("i ref out"=w431:refnum<vi>, "error out"=w432:errorcluster)  [unwired: 12 in, 1 out]
            }
            frame Error {
              n150 = call "CoreLib.set data type mismatch.vi"("error in (no error)"=w437, "error source"=w435) -> ("error out"=w436:errorcluster)  [unwired: 17 in]
            }
          }
          n151 = call "BaseProcess.set event status.vi"("i ref in"=w418, "EventStatus"=w415, "error in (no error)"=w417) -> ("i ref out"=w414:refnum<vi>, "error out"=w416:errorcluster)  [unwired: 14 in, 1 out]
          n152 = case shown="No Error" w416 {
            selector: w416 -> [_ w427]
            tunnel: [_ w426] -> w419
            frame No Error {
            }
            frame Error {
              n153 = Unbundle By Name(w427) -> ("source"=w425:string)
              n154 = call-poly "CoreLib.data 2 byte array.vi"("string"=w425) -> ("byteArray out"=w426:T1)  [unwired: 18 in]
            }
          }
          n155 = Unbundle By Name(w416) -> ("code"=w422:i32)
          n156 = Bundle By Name(cluster=w421, "Data"=w419, "Error #"=w422) -> (w420:T2)
        }
        frame "SetAxisPosition" {
          n157 = Unbundle By Name(w453) -> ("Data"=w445:T1)
          n158 = call-poly "CoreLib.byte array 2 data.vi"("byteArray"=w445) -> ("byteArray out"=w443:T1, "i32"=w441:i32, "error out"=w444:errorcluster)  [unwired: 16 in]
          n159 = call-poly "CoreLib.byte array 2 data.vi"("byteArray"=w443, "error in (no error)"=w444) -> ("d64"=w440:dbl, "error out"=w442:errorcluster)  [unwired: 15 in, 1 out]
          n160 = case shown="No Error" w442 {
            tunnel: [w463 w470] -> w450
            tunnel: w456 -> [w466 w470]
            tunnel: w455 -> [w465 w469]
            tunnel: [w464 w468] -> w449
            tunnel: w440 -> [w461 _]
            tunnel: w447 -> [_ w467]
            tunnel: w441 -> [w462 _]
            tunnel: w439 -> [w460 _]
            frame No Error {
              n161 = call "NanotecSMCPD.set axis position.vi"("i ref in"=w466, "axis"=w462, "position"=w461, "ms timeout (10000)"=w460, "error in (no error)"=w465) -> ("i ref out"=w463:refnum<vi>, "error out"=w464:errorcluster)  [unwired: 12 in, 1 out]
            }
            frame Error {
              n162 = call "CoreLib.set data type mismatch.vi"("error in (no error)"=w469, "error source"=w467) -> ("error out"=w468:errorcluster)  [unwired: 17 in]
            }
          }
          n163 = call "BaseProcess.set event status.vi"("i ref in"=w450, "EventStatus"=w447, "error in (no error)"=w449) -> ("i ref out"=w446:refnum<vi>, "error out"=w448:errorcluster)  [unwired: 14 in, 1 out]
          n164 = case shown="No Error" w448 {
            selector: w448 -> [_ w459]
            tunnel: [_ w458] -> w451
            frame No Error {
            }
            frame Error {
              n165 = Unbundle By Name(w459) -> ("source"=w457:string)
              n166 = call-poly "CoreLib.data 2 byte array.vi"("string"=w457) -> ("byteArray out"=w458:T1)  [unwired: 18 in]
            }
          }
          n167 = Unbundle By Name(w448) -> ("code"=w454:i32)
          n168 = Bundle By Name(cluster=w453, "Data"=w451, "Error #"=w454) -> (w452:T2)
        }
        frame "MoveAxisAbsolute" {
          n169 = Unbundle By Name(w485) -> ("Data"=w477:T1)
          n170 = call-poly "CoreLib.byte array 2 data.vi"("byteArray"=w477) -> ("byteArray out"=w475:T1, "i32"=w473:i32, "error out"=w476:errorcluster)  [unwired: 16 in]
          n171 = call-poly "CoreLib.byte array 2 data.vi"("byteArray"=w475, "error in (no error)"=w476) -> ("d64"=w472:dbl, "error out"=w474:errorcluster)  [unwired: 15 in, 1 out]
          n172 = case shown="No Error" w474 {
            tunnel: [w496 w507] -> w482
            tunnel: w488 -> [w500 w507]
            tunnel: w487 -> [w499 w506]
            tunnel: [w497 w505] -> w481
            tunnel: w472 -> [w495 _]
            tunnel: w479 -> [_ w504]
            tunnel: w473 -> [w494 _]
            tunnel: w471 -> [_ _]
            frame No Error {
              w493 = T5 {"Method"=enum."MoveRelative", "Axis"=0, "Steps"=0.0}  # StoredMethod
              n173 = call "NanotecSMCPD.get i attribute.vi"("i ref in"=w500, "error in (no error)"=w499) -> ("i ref out"=w496:refnum<vi>, "i attribute"=w503:T6, "error out"=w498:errorcluster)  [unwired: 15 in]
              n174 = Unbundle By Name(w503) -> ("MethodQueue"=w502:refnum<queue>)
              n175 = Bundle By Name(cluster=w493, "Method"=enum16{"MoveRelative", "MoveAbsolute", "Stop"}."MoveAbsolute", "Axis"=w494, "Steps"=w495) -> (w501:T5)
              n176 = Lossy Enqueue Element(queue=w502, element=w501, error in (no error)=w498) -> (error out=w497:errorcluster)  [unwired: 3 out]
            }
            frame Error {
              n177 = call "CoreLib.set data type mismatch.vi"("error in (no error)"=w506, "error source"=w504) -> ("error out"=w505:errorcluster)  [unwired: 17 in]
            }
          }
          n178 = call "BaseProcess.set event status.vi"("i ref in"=w482, "EventStatus"=w479, "error in (no error)"=w481) -> ("i ref out"=w478:refnum<vi>, "error out"=w480:errorcluster)  [unwired: 14 in, 1 out]
          n179 = case shown="No Error" w480 {
            selector: w480 -> [_ w491]
            tunnel: [_ w490] -> w483
            frame No Error {
            }
            frame Error {
              n180 = Unbundle By Name(w491) -> ("source"=w489:string)
              n181 = call-poly "CoreLib.data 2 byte array.vi"("string"=w489) -> ("byteArray out"=w490:T1)  [unwired: 18 in]
            }
          }
          n182 = Unbundle By Name(w480) -> ("code"=w486:i32)
          n183 = Bundle By Name(cluster=w485, "Data"=w483, "Error #"=w486) -> (w484:T2)
        }
        frame "MoveAxisRelative" {
          n184 = Unbundle By Name(w522) -> ("Data"=w514:T1)
          n185 = call-poly "CoreLib.byte array 2 data.vi"("byteArray"=w514) -> ("byteArray out"=w512:T1, "i32"=w510:i32, "error out"=w513:errorcluster)  [unwired: 16 in]
          n186 = call-poly "CoreLib.byte array 2 data.vi"("byteArray"=w512, "error in (no error)"=w513) -> ("d64"=w509:dbl, "error out"=w511:errorcluster)  [unwired: 15 in, 1 out]
          n187 = case shown="No Error" w511 {
            tunnel: [w534 w544] -> w519
            tunnel: w525 -> [w537 w544]
            tunnel: w524 -> [w536 w543]
            tunnel: [w533 w542] -> w518
            tunnel: w509 -> [w532 _]
            tunnel: w516 -> [_ w541]
            tunnel: w510 -> [w531 _]
            tunnel: w508 -> [_ _]
            frame No Error {
              w530 = T5 {"Method"=enum."MoveRelative", "Axis"=0, "Steps"=0.0}  # StoredMethod
              n188 = call "NanotecSMCPD.get i attribute.vi"("i ref in"=w537, "error in (no error)"=w536) -> ("i ref out"=w534:refnum<vi>, "i attribute"=w540:T6, "error out"=w535:errorcluster)  [unwired: 15 in]
              n189 = Unbundle By Name(w540) -> ("MethodQueue"=w539:refnum<queue>)
              n190 = Bundle By Name(cluster=w530, "Method"=enum16{"MoveRelative", "MoveAbsolute", "Stop"}."MoveRelative", "Axis"=w531, "Steps"=w532) -> (w538:T5)
              n191 = Lossy Enqueue Element(queue=w539, element=w538, error in (no error)=w535) -> (error out=w533:errorcluster)  [unwired: 3 out]
            }
            frame Error {
              n192 = call "CoreLib.set data type mismatch.vi"("error in (no error)"=w543, "error source"=w541) -> ("error out"=w542:errorcluster)  [unwired: 17 in]
            }
          }
          n193 = call "BaseProcess.set event status.vi"("i ref in"=w519, "EventStatus"=w516, "error in (no error)"=w518) -> ("i ref out"=w515:refnum<vi>, "error out"=w517:errorcluster)  [unwired: 14 in, 1 out]
          n194 = case shown="No Error" w517 {
            selector: w517 -> [_ w528]
            tunnel: [_ w527] -> w520
            frame No Error {
            }
            frame Error {
              n195 = Unbundle By Name(w528) -> ("source"=w526:string)
              n196 = call-poly "CoreLib.data 2 byte array.vi"("string"=w526) -> ("byteArray out"=w527:T1)  [unwired: 18 in]
            }
          }
          n197 = Unbundle By Name(w517) -> ("code"=w523:i32)
          n198 = Bundle By Name(cluster=w522, "Data"=w520, "Error #"=w523) -> (w521:T2)
        }
        frame "Initialize" {
          n199 = Unbundle By Name(w562) -> ("Data"=w553:T1)
          n200 = call-poly "CoreLib.byte array 2 data.vi"("byteArray"=w553) -> ("byteArray out"=w551:T1, "i16"=w549:i16, "error out"=w552:errorcluster)  [unwired: 16 in]
          n201 = call-poly "CoreLib.byte array 2 data.vi"("byteArray"=w551, "error in (no error)"=w552) -> ("i16"=w548:i16, "error out"=w550:errorcluster)  [unwired: 15 in, 1 out]
          n202 = Not Equal To 0?(x=w549) -> (x != 0?=w546:bool)
          n203 = Not Equal To 0?(x=w548) -> (x != 0?=w545:bool)
          n204 = case shown="No Error" w550 {
            tunnel: [w578 w583] -> w559
            tunnel: w566 -> [w579 w583]
            tunnel: w565 -> [w574 w582]
            tunnel: [w573 w581] -> w558
            tunnel: w545 -> [w575 _]
            tunnel: [w572 _] -> w564
            tunnel: w556 -> [_ w580]
            tunnel: w546 -> [w576 _]
            tunnel: w547 -> [w577 _]
            frame No Error {
              n205 = call "NanotecSMCPD.initialize.vi"("i ref in"=w579, "queryID"=w576, "resetControllers"=w575, "ms timeout (10000)"=w577, "error in (no error)"=w574) -> ("i ref out"=w578:refnum<vi>, "deviceID"=w572:string, "error out"=w573:errorcluster)  [unwired: 11 in, 1 out]
            }
            frame Error {
              n206 = call "CoreLib.set data type mismatch.vi"("error in (no error)"=w582, "error source"=w580) -> ("error out"=w581:errorcluster)  [unwired: 17 in]
            }
          }
          n207 = call "BaseProcess.set event status.vi"("i ref in"=w559, "EventStatus"=w556, "error in (no error)"=w558) -> ("i ref out"=w555:refnum<vi>, "error out"=w557:errorcluster)  [unwired: 14 in, 1 out]
          n208 = case shown="No Error" w557 {
            selector: w557 -> [_ w571]
            tunnel: [w567 w570] -> w560
            tunnel: w564 -> [w568 _]
            frame No Error {
              n209 = call-poly "CoreLib.data 2 byte array.vi"("string"=w568) -> ("byteArray out"=w567:T1)  [unwired: 18 in]
            }
            frame Error {
              n210 = Unbundle By Name(w571) -> ("source"=w569:string)
              n211 = call-poly "CoreLib.data 2 byte array.vi"("string"=w569) -> ("byteArray out"=w570:T1)  [unwired: 18 in]
            }
          }
          n212 = Unbundle By Name(w557) -> ("code"=w563:i32)
          n213 = Bundle By Name(cluster=w562, "Data"=w560, "Error #"=w563, "Data Descriptor"="C:N") -> (w561:T2)
        }
        frame "SetStartVelocity" {
          n214 = Unbundle By Name(w595) -> ("Data"=w587:T1)
          n215 = call-poly "CoreLib.byte array 2 data.vi"("byteArray"=w587) -> ("d64"=w584:dbl, "error out"=w585:errorcluster)  [unwired: 16 in, 1 out]
          n216 = case shown="No Error" w585 {
            tunnel: [w610 w614] -> w592
            tunnel: w598 -> [w607 w614]
            tunnel: w597 -> [w606 w613]
            tunnel: [w608 w612] -> w591
            tunnel: w589 -> [_ w611]
            tunnel: w584 -> [w602 _]
            tunnel: w586 -> [w609 _]
            frame No Error {
              n217 = call "MotorBase.get default axis index.vi"("i ref in"=w607, "error in (no error)"=w606) -> ("i ref out"=w604:refnum<vi>, "defaultAxisIndex"=w603:i32, "error out"=w605:errorcluster)  [unwired: 15 in]
              n218 = call "NanotecSMCPD.set axis start velocity.vi"("i ref in"=w604, "axis"=w603, "velocity [units/s]"=w602, "ms timeout (10000)"=w609, "error in (no error)"=w605) -> ("i ref out"=w610:refnum<vi>, "error out"=w608:errorcluster)  [unwired: 12 in, 1 out]
            }
            frame Error {
              n219 = call "CoreLib.set data type mismatch.vi"("error in (no error)"=w613, "error source"=w611) -> ("error out"=w612:errorcluster)  [unwired: 17 in]
            }
          }
          n220 = call "BaseProcess.set event status.vi"("i ref in"=w592, "EventStatus"=w589, "error in (no error)"=w591) -> ("i ref out"=w588:refnum<vi>, "error out"=w590:errorcluster)  [unwired: 14 in, 1 out]
          n221 = case shown="Error" w590 {
            selector: w590 -> [_ w601]
            tunnel: [_ w600] -> w593
            frame No Error {
            }
            frame Error {
              n222 = Unbundle By Name(w601) -> ("source"=w599:string)
              n223 = call-poly "CoreLib.data 2 byte array.vi"("string"=w599) -> ("byteArray out"=w600:T1)  [unwired: 18 in]
            }
          }
          n224 = Unbundle By Name(w590) -> ("code"=w596:i32)
          n225 = Bundle By Name(cluster=w595, "Data"=w593, "Error #"=w596) -> (w594:T2)
        }
        frame "SetStopVelocity" {
          n226 = Unbundle By Name(w626) -> ("Data"=w618:T1)
          n227 = call-poly "CoreLib.byte array 2 data.vi"("byteArray"=w618) -> ("d64"=w615:dbl, "error out"=w616:errorcluster)  [unwired: 16 in, 1 out]
          n228 = case shown="No Error" w616 {
            tunnel: [w641 w645] -> w623
            tunnel: w629 -> [w638 w645]
            tunnel: w628 -> [w637 w644]
            tunnel: [w639 w643] -> w622
            tunnel: w620 -> [_ w642]
            tunnel: w615 -> [w633 _]
            tunnel: w617 -> [w640 _]
            frame No Error {
              n229 = call "MotorBase.get default axis index.vi"("i ref in"=w638, "error in (no error)"=w637) -> ("i ref out"=w635:refnum<vi>, "defaultAxisIndex"=w634:i32, "error out"=w636:errorcluster)  [unwired: 15 in]
              n230 = call "NanotecSMCPD.set axis stop velocity.vi"("i ref in"=w635, "axis"=w634, "velocity [units/s]"=w633, "ms timeout (10000)"=w640, "error in (no error)"=w636) -> ("i ref out"=w641:refnum<vi>, "error out"=w639:errorcluster)  [unwired: 12 in, 1 out]
            }
            frame Error {
              n231 = call "CoreLib.set data type mismatch.vi"("error in (no error)"=w644, "error source"=w642) -> ("error out"=w643:errorcluster)  [unwired: 17 in]
            }
          }
          n232 = call "BaseProcess.set event status.vi"("i ref in"=w623, "EventStatus"=w620, "error in (no error)"=w622) -> ("i ref out"=w619:refnum<vi>, "error out"=w621:errorcluster)  [unwired: 14 in, 1 out]
          n233 = case shown="Error" w621 {
            selector: w621 -> [_ w632]
            tunnel: [_ w631] -> w624
            frame No Error {
            }
            frame Error {
              n234 = Unbundle By Name(w632) -> ("source"=w630:string)
              n235 = call-poly "CoreLib.data 2 byte array.vi"("string"=w630) -> ("byteArray out"=w631:T1)  [unwired: 18 in]
            }
          }
          n236 = Unbundle By Name(w621) -> ("code"=w627:i32)
          n237 = Bundle By Name(cluster=w626, "Data"=w624, "Error #"=w627) -> (w625:T2)
        }
        frame "SetAcceleration" {
          n238 = Unbundle By Name(w657) -> ("Data"=w649:T1)
          n239 = call-poly "CoreLib.byte array 2 data.vi"("byteArray"=w649) -> ("d64"=w646:dbl, "error out"=w647:errorcluster)  [unwired: 16 in, 1 out]
          n240 = case shown="No Error" w647 {
            tunnel: [w672 w676] -> w654
            tunnel: w660 -> [w669 w676]
            tunnel: w659 -> [w668 w675]
            tunnel: [w670 w674] -> w653
            tunnel: w651 -> [_ w673]
            tunnel: w646 -> [w664 _]
            tunnel: w648 -> [w671 _]
            frame No Error {
              n241 = call "MotorBase.get default axis index.vi"("i ref in"=w669, "error in (no error)"=w668) -> ("i ref out"=w666:refnum<vi>, "defaultAxisIndex"=w665:i32, "error out"=w667:errorcluster)  [unwired: 15 in]
              n242 = call "NanotecSMCPD.set axis acceleration.vi"("i ref in"=w666, "axis"=w665, "acceleration [unit/s^2]"=w664, "ms timeout (10000)"=w671, "error in (no error)"=w667) -> ("i ref out"=w672:refnum<vi>, "error out"=w670:errorcluster)  [unwired: 12 in, 1 out]
            }
            frame Error {
              n243 = call "CoreLib.set data type mismatch.vi"("error in (no error)"=w675, "error source"=w673) -> ("error out"=w674:errorcluster)  [unwired: 17 in]
            }
          }
          n244 = call "BaseProcess.set event status.vi"("i ref in"=w654, "EventStatus"=w651, "error in (no error)"=w653) -> ("i ref out"=w650:refnum<vi>, "error out"=w652:errorcluster)  [unwired: 14 in, 1 out]
          n245 = case shown="Error" w652 {
            selector: w652 -> [_ w663]
            tunnel: [_ w662] -> w655
            frame No Error {
            }
            frame Error {
              n246 = Unbundle By Name(w663) -> ("source"=w661:string)
              n247 = call-poly "CoreLib.data 2 byte array.vi"("string"=w661) -> ("byteArray out"=w662:T1)  [unwired: 18 in]
            }
          }
          n248 = Unbundle By Name(w652) -> ("code"=w658:i32)
          n249 = Bundle By Name(cluster=w657, "Data"=w655, "Error #"=w658) -> (w656:T2)
        }
        frame "SetPosition" {
          n250 = Unbundle By Name(w688) -> ("Data"=w680:T1)
          n251 = call-poly "CoreLib.byte array 2 data.vi"("byteArray"=w680) -> ("d64"=w677:dbl, "error out"=w678:errorcluster)  [unwired: 16 in, 1 out]
          n252 = case shown="No Error" w678 {
            tunnel: [w703 w707] -> w685
            tunnel: w691 -> [w700 w707]
            tunnel: w690 -> [w699 w706]
            tunnel: [w701 w705] -> w684
            tunnel: w682 -> [_ w704]
            tunnel: w677 -> [w695 _]
            tunnel: w679 -> [w702 _]
            frame No Error {
              n253 = call "MotorBase.get default axis index.vi"("i ref in"=w700, "error in (no error)"=w699) -> ("i ref out"=w697:refnum<vi>, "defaultAxisIndex"=w696:i32, "error out"=w698:errorcluster)  [unwired: 15 in]
              n254 = call "NanotecSMCPD.set axis position.vi"("i ref in"=w697, "axis"=w696, "position"=w695, "ms timeout (10000)"=w702, "error in (no error)"=w698) -> ("i ref out"=w703:refnum<vi>, "error out"=w701:errorcluster)  [unwired: 12 in, 1 out]
            }
            frame Error {
              n255 = call "CoreLib.set data type mismatch.vi"("error in (no error)"=w706, "error source"=w704) -> ("error out"=w705:errorcluster)  [unwired: 17 in]
            }
          }
          n256 = call "BaseProcess.set event status.vi"("i ref in"=w685, "EventStatus"=w682, "error in (no error)"=w684) -> ("i ref out"=w681:refnum<vi>, "error out"=w683:errorcluster)  [unwired: 14 in, 1 out]
          n257 = case shown="Error" w683 {
            selector: w683 -> [_ w694]
            tunnel: [_ w693] -> w686
            frame No Error {
            }
            frame Error {
              n258 = Unbundle By Name(w694) -> ("source"=w692:string)
              n259 = call-poly "CoreLib.data 2 byte array.vi"("string"=w692) -> ("byteArray out"=w693:T1)  [unwired: 18 in]
            }
          }
          n260 = Unbundle By Name(w683) -> ("code"=w689:i32)
          n261 = Bundle By Name(cluster=w688, "Data"=w686, "Error #"=w689) -> (w687:T2)
        }
        frame "MoveAbsolute" {
          n262 = Unbundle By Name(w719) -> ("Data"=w711:T1)
          n263 = call-poly "CoreLib.byte array 2 data.vi"("byteArray"=w711) -> ("d64"=w708:dbl, "error out"=w709:errorcluster)  [unwired: 16 in, 1 out]
          n264 = case shown="No Error" w709 {
            tunnel: [w730 w743] -> w716
            tunnel: w722 -> [w739 w743]
            tunnel: w721 -> [w738 w742]
            tunnel: [w731 w741] -> w715
            tunnel: w713 -> [_ w740]
            tunnel: w708 -> [w729 _]
            tunnel: w710 -> [_ _]
            frame No Error {
              w727 = T5 {"Method"=enum."MoveRelative", "Axis"=0, "Steps"=0.0}  # StoredMethod
              n265 = call "MotorBase.get default axis index.vi"("i ref in"=w739, "error in (no error)"=w738) -> ("i ref out"=w734:refnum<vi>, "defaultAxisIndex"=w728:i32, "error out"=w733:errorcluster)  [unwired: 15 in]
              n266 = call "NanotecSMCPD.get i attribute.vi"("i ref in"=w734, "error in (no error)"=w733) -> ("i ref out"=w730:refnum<vi>, "i attribute"=w737:T6, "error out"=w732:errorcluster)  [unwired: 15 in]
              n267 = Unbundle By Name(w737) -> ("MethodQueue"=w736:refnum<queue>)
              n268 = Bundle By Name(cluster=w727, "Method"=enum16{"MoveRelative", "MoveAbsolute", "Stop"}."MoveAbsolute", "Axis"=w728, "Steps"=w729) -> (w735:T5)
              n269 = Lossy Enqueue Element(queue=w736, element=w735, error in (no error)=w732) -> (error out=w731:errorcluster)  [unwired: 3 out]
            }
            frame Error {
              n270 = call "CoreLib.set data type mismatch.vi"("error in (no error)"=w742, "error source"=w740) -> ("error out"=w741:errorcluster)  [unwired: 17 in]
            }
          }
          n271 = call "BaseProcess.set event status.vi"("i ref in"=w716, "EventStatus"=w713, "error in (no error)"=w715) -> ("i ref out"=w712:refnum<vi>, "error out"=w714:errorcluster)  [unwired: 14 in, 1 out]
          n272 = case shown="Error" w714 {
            selector: w714 -> [_ w725]
            tunnel: [_ w724] -> w717
            frame No Error {
            }
            frame Error {
              n273 = Unbundle By Name(w725) -> ("source"=w723:string)
              n274 = call-poly "CoreLib.data 2 byte array.vi"("string"=w723) -> ("byteArray out"=w724:T1)  [unwired: 18 in]
            }
          }
          n275 = Unbundle By Name(w714) -> ("code"=w720:i32)
          n276 = Bundle By Name(cluster=w719, "Data"=w717, "Error #"=w720) -> (w718:T2)
        }
        frame "MoveRelative" {
          n277 = Unbundle By Name(w755) -> ("Data"=w747:T1)
          n278 = call-poly "CoreLib.byte array 2 data.vi"("byteArray"=w747) -> ("d64"=w744:dbl, "error out"=w745:errorcluster)  [unwired: 16 in, 1 out]
          n279 = case shown="No Error" w745 {
            tunnel: [w766 w779] -> w752
            tunnel: w758 -> [w775 w779]
            tunnel: w757 -> [w774 w778]
            tunnel: [w767 w777] -> w751
            tunnel: w749 -> [_ w776]
            tunnel: w744 -> [w764 _]
            tunnel: w746 -> [_ _]
            frame No Error {
              w763 = T5 {"Method"=enum."MoveRelative", "Axis"=0, "Steps"=0.0}  # StoredMethod
              n280 = call "MotorBase.get default axis index.vi"("i ref in"=w775, "error in (no error)"=w774) -> ("i ref out"=w770:refnum<vi>, "defaultAxisIndex"=w765:i32, "error out"=w769:errorcluster)  [unwired: 15 in]
              n281 = call "NanotecSMCPD.get i attribute.vi"("i ref in"=w770, "error in (no error)"=w769) -> ("i ref out"=w766:refnum<vi>, "i attribute"=w771:T6, "error out"=w768:errorcluster)  [unwired: 15 in]
              n282 = Unbundle By Name(w771) -> ("MethodQueue"=w772:refnum<queue>)
              n283 = Bundle By Name(cluster=w763, "Method"=enum16{"MoveRelative", "MoveAbsolute", "Stop"}."MoveRelative", "Axis"=w765, "Steps"=w764) -> (w773:T5)
              n284 = Lossy Enqueue Element(queue=w772, element=w773, error in (no error)=w768) -> (error out=w767:errorcluster)  [unwired: 3 out]
            }
            frame Error {
              n285 = call "CoreLib.set data type mismatch.vi"("error in (no error)"=w778, "error source"=w776) -> ("error out"=w777:errorcluster)  [unwired: 17 in]
            }
          }
          n286 = call "BaseProcess.set event status.vi"("i ref in"=w752, "EventStatus"=w749, "error in (no error)"=w751) -> ("i ref out"=w748:refnum<vi>, "error out"=w750:errorcluster)  [unwired: 14 in, 1 out]
          n287 = case shown="Error" w750 {
            selector: w750 -> [_ w761]
            tunnel: [_ w760] -> w753
            frame No Error {
            }
            frame Error {
              n288 = Unbundle By Name(w761) -> ("source"=w759:string)
              n289 = call-poly "CoreLib.data 2 byte array.vi"("string"=w759) -> ("byteArray out"=w760:T1)  [unwired: 18 in]
            }
          }
          n290 = Unbundle By Name(w750) -> ("code"=w756:i32)
          n291 = Bundle By Name(cluster=w755, "Data"=w753, "Error #"=w756) -> (w754:T2)
        }
        frame "GetStartVelocity" {
          n292 = call "MotorBase.get default axis index.vi"("i ref in"=w796, "error in (no error)"=w795) -> ("i ref out"=w783:refnum<vi>, "defaultAxisIndex"=w782:i32, "error out"=w784:errorcluster)  [unwired: 15 in]
          n293 = call "NanotecSMCPD.get axis start velocity.vi"("i ref in"=w783, "axis"=w782, "ms timeout (10000)"=w785, "error in (no error)"=w784) -> ("i ref out"=w790:refnum<vi>, "startVelocity [unit/s]"=w781:dbl, "error out"=w789:errorcluster)  [unwired: 12 in, 1 out]
          n294 = call "BaseProcess.set event status.vi"("i ref in"=w790, "EventStatus"=w787, "error in (no error)"=w789) -> ("i ref out"=w786:refnum<vi>, "error out"=w788:errorcluster)  [unwired: 14 in, 1 out]
          n295 = case shown="No Error" w788 {
            selector: w788 -> [_ w801]
            tunnel: [w798 w800] -> w791
            tunnel: w781 -> [w797 _]
            frame No Error {
              n296 = call-poly "CoreLib.data 2 byte array.vi"("f64"=w797) -> ("byteArray out"=w798:T1)  [unwired: 18 in]
            }
            frame Error {
              n297 = Unbundle By Name(w801) -> ("source"=w799:string)
              n298 = call-poly "CoreLib.data 2 byte array.vi"("string"=w799) -> ("byteArray out"=w800:T1)  [unwired: 18 in]
            }
          }
          n299 = Unbundle By Name(w788) -> ("code"=w794:i32)
          n300 = Bundle By Name(cluster=w793, "Data"=w791, "Error #"=w794, "Data Descriptor"=T3 "D:1") -> (w792:T2)
        }
        frame "GetStopVelocity" {
          n301 = call "MotorBase.get default axis index.vi"("i ref in"=w818, "error in (no error)"=w817) -> ("i ref out"=w805:refnum<vi>, "defaultAxisIndex"=w804:i32, "error out"=w806:errorcluster)  [unwired: 15 in]
          n302 = call "NanotecSMCPD.get axis stop velocity.vi"("i ref in"=w805, "axis"=w804, "ms timeout (10000)"=w807, "error in (no error)"=w806) -> ("i ref out"=w812:refnum<vi>, "stopVelocity [unit/s]"=w803:dbl, "error out"=w811:errorcluster)  [unwired: 12 in, 1 out]
          n303 = call "BaseProcess.set event status.vi"("i ref in"=w812, "EventStatus"=w809, "error in (no error)"=w811) -> ("i ref out"=w808:refnum<vi>, "error out"=w810:errorcluster)  [unwired: 14 in, 1 out]
          n304 = case shown="No Error" w810 {
            selector: w810 -> [_ w823]
            tunnel: [w820 w822] -> w813
            tunnel: w803 -> [w819 _]
            frame No Error {
              n305 = call-poly "CoreLib.data 2 byte array.vi"("f64"=w819) -> ("byteArray out"=w820:T1)  [unwired: 18 in]
            }
            frame Error {
              n306 = Unbundle By Name(w823) -> ("source"=w821:string)
              n307 = call-poly "CoreLib.data 2 byte array.vi"("string"=w821) -> ("byteArray out"=w822:T1)  [unwired: 18 in]
            }
          }
          n308 = Unbundle By Name(w810) -> ("code"=w816:i32)
          n309 = Bundle By Name(cluster=w815, "Data"=w813, "Error #"=w816, "Data Descriptor"=T3 "D:1") -> (w814:T2)
        }
        frame "GetAcceleration" {
          n310 = call "MotorBase.get default axis index.vi"("i ref in"=w840, "error in (no error)"=w839) -> ("i ref out"=w827:refnum<vi>, "defaultAxisIndex"=w826:i32, "error out"=w828:errorcluster)  [unwired: 15 in]
          n311 = call "NanotecSMCPD.get axis acceleration.vi"("i ref in"=w827, "axis"=w826, "ms timeout (10000)"=w829, "error in (no error)"=w828) -> ("i ref out"=w834:refnum<vi>, "acceleration [unit/s^2]"=w825:dbl, "error out"=w833:errorcluster)  [unwired: 12 in, 1 out]
          n312 = call "BaseProcess.set event status.vi"("i ref in"=w834, "EventStatus"=w831, "error in (no error)"=w833) -> ("i ref out"=w830:refnum<vi>, "error out"=w832:errorcluster)  [unwired: 14 in, 1 out]
          n313 = case shown="No Error" w832 {
            selector: w832 -> [_ w845]
            tunnel: [w842 w844] -> w835
            tunnel: w825 -> [w841 _]
            frame No Error {
              n314 = call-poly "CoreLib.data 2 byte array.vi"("f64"=w841) -> ("byteArray out"=w842:T1)  [unwired: 18 in]
            }
            frame Error {
              n315 = Unbundle By Name(w845) -> ("source"=w843:string)
              n316 = call-poly "CoreLib.data 2 byte array.vi"("string"=w843) -> ("byteArray out"=w844:T1)  [unwired: 18 in]
            }
          }
          n317 = Unbundle By Name(w832) -> ("code"=w838:i32)
          n318 = Bundle By Name(cluster=w837, "Data"=w835, "Error #"=w838, "Data Descriptor"=T3 "D:1") -> (w836:T2)
        }
        frame "GetPosition" {
          n319 = call "MotorBase.get default axis index.vi"("i ref in"=w862, "error in (no error)"=w861) -> ("i ref out"=w849:refnum<vi>, "defaultAxisIndex"=w848:i32, "error out"=w850:errorcluster)  [unwired: 15 in]
          n320 = call "NanotecSMCPD.get axis position.vi"("i ref in"=w849, "axis"=w848, "ms timeout (10000)"=w851, "error in (no error)"=w850) -> ("i ref out"=w856:refnum<vi>, "position [unit]"=w847:dbl, "error out"=w855:errorcluster)  [unwired: 12 in, 1 out]
          n321 = call "BaseProcess.set event status.vi"("i ref in"=w856, "EventStatus"=w853, "error in (no error)"=w855) -> ("i ref out"=w852:refnum<vi>, "error out"=w854:errorcluster)  [unwired: 14 in, 1 out]
          n322 = case shown="No Error" w854 {
            selector: w854 -> [_ w867]
            tunnel: [w864 w866] -> w857
            tunnel: w847 -> [w863 _]
            frame No Error {
              n323 = call-poly "CoreLib.data 2 byte array.vi"("f64"=w863) -> ("byteArray out"=w864:T1)  [unwired: 18 in]
            }
            frame Error {
              n324 = Unbundle By Name(w867) -> ("source"=w865:string)
              n325 = call-poly "CoreLib.data 2 byte array.vi"("string"=w865) -> ("byteArray out"=w866:T1)  [unwired: 18 in]
            }
          }
          n326 = Unbundle By Name(w854) -> ("code"=w860:i32)
          n327 = Bundle By Name(cluster=w859, "Data"=w857, "Error #"=w860, "Data Descriptor"=T3 "D:1") -> (w858:T2)
        }
        frame "GetStatus" {
          n328 = call "MotorBase.get default axis index.vi"("i ref in"=w884, "error in (no error)"=w883) -> ("i ref out"=w871:refnum<vi>, "defaultAxisIndex"=w870:i32, "error out"=w872:errorcluster)  [unwired: 15 in]
          n329 = call "NanotecSMCPD.get axis status.vi"("i ref in"=w871, "axis"=w870, "ms timeout (10000)"=w873, "error in (no error)"=w872) -> ("i ref out"=w878:refnum<vi>, "status"=w869:T4, "error out"=w877:errorcluster)  [unwired: 11 in, 2 out]
          n330 = call "BaseProcess.set event status.vi"("i ref in"=w878, "EventStatus"=w875, "error in (no error)"=w877) -> ("i ref out"=w874:refnum<vi>, "error out"=w876:errorcluster)  [unwired: 14 in, 1 out]
          n331 = case shown="No Error" w876 {
            selector: w876 -> [_ w890]
            tunnel: [w887 w889] -> w879
            tunnel: w869 -> [w886 _]
            frame No Error {
              n332 = To Long Integer(number=w886) -> (32bit integer=w885:i32)
              n333 = call-poly "CoreLib.data 2 byte array.vi"("i32"=w885) -> ("byteArray out"=w887:T1)  [unwired: 18 in]
            }
            frame Error {
              n334 = Unbundle By Name(w890) -> ("source"=w888:string)
              n335 = call-poly "CoreLib.data 2 byte array.vi"("string"=w888) -> ("byteArray out"=w889:T1)  [unwired: 18 in]
            }
          }
          n336 = Unbundle By Name(w876) -> ("code"=w882:i32)
          n337 = Bundle By Name(cluster=w881, "Data"=w879, "Error #"=w882, "Data Descriptor"=T3 "I:1") -> (w880:T2)
        }
        frame "ResetDefault" {
          n338 = call "MotorBase.get default axis index.vi"("i ref in"=w905, "error in (no error)"=w904) -> ("i ref out"=w892:refnum<vi>, "defaultAxisIndex"=w891:i32, "error out"=w893:errorcluster)  [unwired: 15 in]
          n339 = call "NanotecSMCPD.reset axis.vi"("i ref in"=w892, "axis"=w891, "ms timeout (10000)"=w894, "error in (no error)"=w893) -> ("i ref out"=w899:refnum<vi>, "error out"=w898:errorcluster)  [unwired: 13 in, 1 out]
          n340 = call "BaseProcess.set event status.vi"("i ref in"=w899, "EventStatus"=w896, "error in (no error)"=w898) -> ("i ref out"=w895:refnum<vi>, "error out"=w897:errorcluster)  [unwired: 14 in, 1 out]
          n341 = case shown="No Error" w897 {
            selector: w897 -> [_ w908]
            tunnel: [_ w907] -> w900
            frame No Error {
            }
            frame Error {
              n342 = Unbundle By Name(w908) -> ("source"=w906:string)
              n343 = call-poly "CoreLib.data 2 byte array.vi"("string"=w906) -> ("byteArray out"=w907:T1)  [unwired: 18 in]
            }
          }
          n344 = Unbundle By Name(w897) -> ("code"=w903:i32)
          n345 = Bundle By Name(cluster=w902, "Data"=w900, "Error #"=w903) -> (w901:T2)
        }
        frame "FindReference" {
          n346 = call "MotorBase.get default axis index.vi"("i ref in"=w923, "error in (no error)"=w922) -> ("i ref out"=w910:refnum<vi>, "defaultAxisIndex"=w909:i32, "error out"=w911:errorcluster)  [unwired: 15 in]
          n347 = call "NanotecSMCPD.find axis reference.vi"("i ref in"=w910, "axis"=w909, "ms timeout (10000)"=w912, "error in (no error)"=w911) -> ("i ref out"=w917:refnum<vi>, "error out"=w916:errorcluster)  [unwired: 13 in, 1 out]
          n348 = call "BaseProcess.set event status.vi"("i ref in"=w917, "EventStatus"=w914, "error in (no error)"=w916) -> ("i ref out"=w913:refnum<vi>, "error out"=w915:errorcluster)  [unwired: 14 in, 1 out]
          n349 = case shown="No Error" w915 {
            selector: w915 -> [_ w926]
            tunnel: [_ w925] -> w918
            frame No Error {
            }
            frame Error {
              n350 = Unbundle By Name(w926) -> ("source"=w924:string)
              n351 = call-poly "CoreLib.data 2 byte array.vi"("string"=w924) -> ("byteArray out"=w925:T1)  [unwired: 18 in]
            }
          }
          n352 = Unbundle By Name(w915) -> ("code"=w921:i32)
          n353 = Bundle By Name(cluster=w920, "Data"=w918, "Error #"=w921) -> (w919:T2)
        }
        frame "Halt" {
          n354 = call "MotorBase.get default axis index.vi"("i ref in"=w941, "error in (no error)"=w940) -> ("i ref out"=w928:refnum<vi>, "defaultAxisIndex"=w927:i32, "error out"=w929:errorcluster)  [unwired: 15 in]
          n355 = call "NanotecSMCPD.halt axis.vi"("i ref in"=w928, "axis"=w927, "ms timeout (10000)"=w930, "error in (no error)"=w929) -> ("i ref out"=w935:refnum<vi>, "error out"=w934:errorcluster)  [unwired: 13 in, 1 out]
          n356 = call "BaseProcess.set event status.vi"("i ref in"=w935, "EventStatus"=w932, "error in (no error)"=w934) -> ("i ref out"=w931:refnum<vi>, "error out"=w933:errorcluster)  [unwired: 14 in, 1 out]
          n357 = case shown="No Error" w933 {
            selector: w933 -> [_ w944]
            tunnel: [_ w943] -> w936
            frame No Error {
            }
            frame Error {
              n358 = Unbundle By Name(w944) -> ("source"=w942:string)
              n359 = call-poly "CoreLib.data 2 byte array.vi"("string"=w942) -> ("byteArray out"=w943:T1)  [unwired: 18 in]
            }
          }
          n360 = Unbundle By Name(w933) -> ("code"=w939:i32)
          n361 = Bundle By Name(cluster=w938, "Data"=w936, "Error #"=w939) -> (w937:T2)
        }
        frame "Close" {
          n362 = call "NanotecSMCPD.close.vi"("i ref in"=w955, "error in (no error)"=w954) -> ("i ref out"=w949:refnum<vi>, "error out"=w948:errorcluster)  [unwired: 16 in]
          n363 = call "BaseProcess.set event status.vi"("i ref in"=w949, "EventStatus"=w946, "error in (no error)"=w948) -> ("i ref out"=w945:refnum<vi>, "error out"=w947:errorcluster)  [unwired: 14 in, 1 out]
          n364 = case shown="No Error" w947 {
            selector: w947 -> [_ w958]
            tunnel: [_ w957] -> w950
            frame No Error {
            }
            frame Error {
              n365 = Unbundle By Name(w958) -> ("source"=w956:string)
              n366 = call-poly "CoreLib.data 2 byte array.vi"("string"=w956) -> ("byteArray out"=w957:T1)  [unwired: 18 in]
            }
          }
          n367 = Unbundle By Name(w947) -> ("code"=w953:i32)
          n368 = Bundle By Name(cluster=w952, "Data"=w950, "Error #"=w953) -> (w951:T2)
        }
        frame "Reset" {
          n369 = call "NanotecSMCPD.reset.vi"("i ref in"=w970, "ms timeout (10000)"=w959, "error in (no error)"=w969) -> ("i ref out"=w964:refnum<vi>, "error out"=w963:errorcluster)  [unwired: 14 in, 1 out]
          n370 = call "BaseProcess.set event status.vi"("i ref in"=w964, "EventStatus"=w961, "error in (no error)"=w963) -> ("i ref out"=w960:refnum<vi>, "error out"=w962:errorcluster)  [unwired: 14 in, 1 out]
          n371 = case shown="No Error" w962 {
            selector: w962 -> [_ w973]
            tunnel: [_ w972] -> w965
            frame No Error {
            }
            frame Error {
              n372 = Unbundle By Name(w973) -> ("source"=w971:string)
              n373 = call-poly "CoreLib.data 2 byte array.vi"("string"=w971) -> ("byteArray out"=w972:T1)  [unwired: 18 in]
            }
          }
          n374 = Unbundle By Name(w962) -> ("code"=w968:i32)
          n375 = Bundle By Name(cluster=w967, "Data"=w965, "Error #"=w968) -> (w966:T2)
        }
        frame "IDQuery" {
          n376 = call "NanotecSMCPD.ID query.vi"("i ref in"=w987, "ms timeout (10000)"=w976, "error in (no error)"=w986) -> ("i ref out"=w981:refnum<vi>, "deviceID"=w975:string, "error out"=w980:errorcluster)  [unwired: 13 in, 1 out]
          n377 = call "BaseProcess.set event status.vi"("i ref in"=w981, "EventStatus"=w978, "error in (no error)"=w980) -> ("i ref out"=w977:refnum<vi>, "error out"=w979:errorcluster)  [unwired: 14 in, 1 out]
          n378 = case shown="No Error" w979 {
            selector: w979 -> [_ w992]
            tunnel: [w989 w991] -> w982
            tunnel: w975 -> [w988 _]
            frame No Error {
              n379 = call-poly "CoreLib.data 2 byte array.vi"("string"=w988) -> ("byteArray out"=w989:T1)  [unwired: 18 in]
            }
            frame Error {
              n380 = Unbundle By Name(w992) -> ("source"=w990:string)
              n381 = call-poly "CoreLib.data 2 byte array.vi"("string"=w990) -> ("byteArray out"=w991:T1)  [unwired: 18 in]
            }
          }
          n382 = Unbundle By Name(w979) -> ("code"=w985:i32)
          n383 = Bundle By Name(cluster=w984, "Data"=w982, "Error #"=w985, "Data Descriptor"=T3 "C:N") -> (w983:T2)
        }
        frame "GetOnOff" {
          n384 = call "MotorBase.get default axis index.vi"("i ref in"=w998, "error in (no error)"=w995) -> ("i ref out"=w996:refnum<vi>, "defaultAxisIndex"=w997:i32, "error out"=w994:errorcluster)  [unwired: 15 in]
          n385 = call "NanotecSMCPD.get axis onOff.vi"("i ref in"=w996, "axis"=w997, "ms timeout (10000)"=w993, "error in (no error)"=w994) -> ("i ref out"=w1007:refnum<vi>, "onOff"=w1002:bool, "error out"=w1006:errorcluster)  [unwired: 12 in, 1 out]
          n386 = Boolean To (0,1)(Boolean=w1002) -> (0, 1=w1001:i16)
          n387 = To Word Integer(number=w1001) -> (16bit integer=w1000:i16)
          n388 = call "BaseProcess.set event status.vi"("i ref in"=w1007, "EventStatus"=w1004, "error in (no error)"=w1006) -> ("i ref out"=w1003:refnum<vi>, "error out"=w1005:errorcluster)  [unwired: 14 in, 1 out]
          n389 = case shown="No Error" w1005 {
            selector: w1005 -> [_ w1016]
            tunnel: [w1013 w1015] -> w1008
            tunnel: w1000 -> [w1012 _]
            frame No Error {
              n390 = call-poly "CoreLib.data 2 byte array.vi"("i16"=w1012) -> ("byteArray out"=w1013:T1)  [unwired: 18 in]
            }
            frame Error {
              n391 = Unbundle By Name(w1016) -> ("source"=w1014:string)
              n392 = call-poly "CoreLib.data 2 byte array.vi"("string"=w1014) -> ("byteArray out"=w1015:T1)  [unwired: 18 in]
            }
          }
          n393 = Unbundle By Name(w1005) -> ("code"=w1011:i32)
          n394 = Bundle By Name(cluster=w1010, "Data"=w1008, "Error #"=w1011, "Data Descriptor"=T3 "S:1") -> (w1009:T2)
        }
        frame "GetAxisOnOff" {
          n395 = Unbundle By Name(w1021) -> ("Data"=w1022:T1)
          n396 = call-poly "CoreLib.byte array 2 data.vi"("byteArray"=w1022) -> ("i32"=w1017:i32, "error out"=w1020:errorcluster)  [unwired: 16 in, 1 out]
          n397 = case shown="No Error" w1020 {
            tunnel: [w1042 w1043] -> w1030
            tunnel: [w1041 w1045] -> w1029
            tunnel: [w1038 _] -> w1026
            tunnel: w1024 -> [w1037 _]
            tunnel: w1023 -> [w1036 w1043]
            tunnel: w1019 -> [w1035 w1046]
            tunnel: w1018 -> [_ w1044]
            tunnel: w1017 -> [w1034 _]
            frame No Error {
              n398 = call "NanotecSMCPD.get axis onOff.vi"("i ref in"=w1036, "axis"=w1034, "ms timeout (10000)"=w1037, "error in (no error)"=w1035) -> ("i ref out"=w1042:refnum<vi>, "onOff"=w1040:bool, "error out"=w1041:errorcluster)  [unwired: 12 in, 1 out]
              n399 = Boolean To (0,1)(Boolean=w1040) -> (0, 1=w1039:i16)
              n400 = To Word Integer(number=w1039) -> (16bit integer=w1038:i16)
            }
            frame Error {
              n401 = call "CoreLib.set data type mismatch.vi"("error in (no error)"=w1046, "error source"=w1044) -> ("error out"=w1045:errorcluster)  [unwired: 17 in]
            }
          }
          n402 = call "BaseProcess.set event status.vi"("i ref in"=w1030, "EventStatus"=w1018, "error in (no error)"=w1029) -> ("i ref out"=w1027:refnum<vi>, "error out"=w1028:errorcluster)  [unwired: 14 in, 1 out]
          n403 = case shown="No Error" w1028 {
            selector: w1028 -> [_ w1051]
            tunnel: [w1048 w1050] -> w1031
            tunnel: w1026 -> [w1047 _]
            frame No Error {
              n404 = call-poly "CoreLib.data 2 byte array.vi"("i16"=w1047) -> ("byteArray out"=w1048:T1)  [unwired: 18 in]
            }
            frame Error {
              n405 = Unbundle By Name(w1051) -> ("source"=w1049:string)
              n406 = call-poly "CoreLib.data 2 byte array.vi"("string"=w1049) -> ("byteArray out"=w1050:T1)  [unwired: 18 in]
            }
          }
          n407 = Unbundle By Name(w1028) -> ("code"=w1033:i32)
          n408 = Bundle By Name(cluster=w1021, "Data"=w1031, "Error #"=w1033, "Data Descriptor"=T3 "S:1") -> (w1032:T2)
        }
        frame "EmergencyOff" {
          n409 = call "NanotecSMCPD.emergency off.vi"("i ref in"=w1056, "ms timeout (10000)"=w1052, "error in (no error)"=w1053) -> ("i ref out"=w1055:refnum<vi>, "error out"=w1054:errorcluster)  [unwired: 14 in, 1 out]
          n410 = call "BaseProcess.set event status.vi"("i ref in"=w1055, "EventStatus"=w1058, "error in (no error)"=w1054) -> ("i ref out"=w1057:refnum<vi>, "error out"=w1059:errorcluster)  [unwired: 14 in, 1 out]
          n411 = case shown="No Error" w1059 {
            selector: w1059 -> [_ w1066]
            tunnel: [_ w1065] -> w1060
            frame No Error {
            }
            frame Error {
              n412 = Unbundle By Name(w1066) -> ("source"=w1064:string)
              n413 = call-poly "CoreLib.data 2 byte array.vi"("string"=w1064) -> ("byteArray out"=w1065:T1)  [unwired: 18 in]
            }
          }
          n414 = Unbundle By Name(w1059) -> ("code"=w1063:i32)
          n415 = Bundle By Name(cluster=w1062, "Data"=w1060, "Error #"=w1063) -> (w1061:T2)
        }
      }
    }
    frame Error {
    }
  }
  "answer cluster" <- w8
  "i ref out" <- w4
  "error out" <- w3
